vi "AluFlon Calibration.vi"() -> ()   [LabVIEW 2020]
uses:
  <vilib>/Instr/_visa.llb/VISA Find Search Mode.ctl
  <vilib>/Utility/miscctls.llb/LVRangeTypeDef.ctl
  de5aae1c-766f-4be6-99a3-fd4ec51816d1.vi
  444d9fc6-818c-47ea-bc58-0d0404dcb872.vi
  b5a75377-d0a3-43d6-8795-20c953c640ae.vi
  d5915287-11e6-429c-9896-de3842618b98.vi
  0cc29e98-fdb5-409f-a0e8-e594b8d976c3.vi
  0322f161-1cbb-43ba-a316-90f580a35a69.vi
  6005b055-fe01-43f0-bd4e-c0c49bb95745.vi
  ecbb4e81-cdd6-4c90-bb4c-f1c9c07fb26c.vi
  1a033c88-510c-45da-922e-66e902a61d4e.vi
  93b92521-9e16-4e93-a709-63335b20948f.vi
  31527b8b-dd2e-4aef-8780-3661b63cca63.vi
  b0d12dfb-2fe3-4095-91e7-f81a6dcb1a5e.vi
  c511048d-5316-4b7a-a317-28d3a9e40be0.vi
  e6c7d1cb-2e94-4559-8f57-83b39ddeefc4.vi
  0a39aaed-6fe6-4517-8bcb-3b5a94f10ea5.vi
  26b90bb2-1f84-4233-ae15-16fa66b975c9.vi
  89507e17-66a2-42ab-9a6b-fa3baa268747.vi
  6f735820-b968-40fe-8dcc-9caa75eabf9b.vi
  379c9800-c512-4a9e-8fef-dcae08926fd9.vi
  6bee6147-41c9-44c0-82a1-e9b70bc37061.vi
  dbb8d4b4-432b-4aa2-b5ee-fb03dd486db5.vi
  9e6f70b0-763e-423b-96ef-59fb8772dfa3.vi
  9a42ad8e-034c-4bb5-99e1-dddd59a1f9b6.vi
  3a4bb5ac-5c5c-4d63-87bf-9b8807b4be2b.vi
  a7842cd6-eb29-4009-89cc-97ffd3691122.vi
  a0a268c4-e710-4790-b893-111d5180be5d.vi
  66df6cea-0bd2-48ae-885a-3d43a00be0e6.vi
  87e030aa-6b8c-4722-a122-ccb5b3d7d58b.vi
  107db427-7959-46f3-9e7b-819df6104af8.vi
  de5aae1c-766f-4be6-99a3-fd4ec51816d1.vi/393b2312-c94a-42b8-a7f2-b1ce51657457.vi
  444d9fc6-818c-47ea-bc58-0d0404dcb872.vi/393b2312-c94a-42b8-a7f2-b1ce51657457.vi
  ecbb4e81-cdd6-4c90-bb4c-f1c9c07fb26c.vi/393b2312-c94a-42b8-a7f2-b1ce51657457.vi
  1a033c88-510c-45da-922e-66e902a61d4e.vi/393b2312-c94a-42b8-a7f2-b1ce51657457.vi
  93b92521-9e16-4e93-a709-63335b20948f.vi/393b2312-c94a-42b8-a7f2-b1ce51657457.vi
  31527b8b-dd2e-4aef-8780-3661b63cca63.vi/393b2312-c94a-42b8-a7f2-b1ce51657457.vi
  b0d12dfb-2fe3-4095-91e7-f81a6dcb1a5e.vi/393b2312-c94a-42b8-a7f2-b1ce51657457.vi
  c511048d-5316-4b7a-a317-28d3a9e40be0.vi/393b2312-c94a-42b8-a7f2-b1ce51657457.vi
  e6c7d1cb-2e94-4559-8f57-83b39ddeefc4.vi/393b2312-c94a-42b8-a7f2-b1ce51657457.vi
  0a39aaed-6fe6-4517-8bcb-3b5a94f10ea5.vi/393b2312-c94a-42b8-a7f2-b1ce51657457.vi
  26b90bb2-1f84-4233-ae15-16fa66b975c9.vi/393b2312-c94a-42b8-a7f2-b1ce51657457.vi
  89507e17-66a2-42ab-9a6b-fa3baa268747.vi/393b2312-c94a-42b8-a7f2-b1ce51657457.vi
  6f735820-b968-40fe-8dcc-9caa75eabf9b.vi/393b2312-c94a-42b8-a7f2-b1ce51657457.vi
  a0a268c4-e710-4790-b893-111d5180be5d.vi/393b2312-c94a-42b8-a7f2-b1ce51657457.vi
  <vilib>/NI Modbus.llb/MB Serial Master Query (poly).vi
  SubVI/MB Serial Master Query Write Single Register (poly).vi
  <vilib>/Utility/file.llb/Write Delimited Spreadsheet (string).vi
  <vilib>/Utility/miscctls.llb/LVStringsAndValuesArrayTypeDef_U16.ctl
panel:
  out "ConnectionFlag":bool=TRUE
  out "Blank Bottom":bool
  in  "visibleArray":bool[](array[boolean])
  in  "ClearTGraph 2":bool caption="Clear"
  in  "Dirt Calibr":bool caption="IRTimeSet"
  in  "ServiceWin":bool
  in  "file path (dialog if empty)":path
  out "Blank Top":bool
  out "FirmW":u16
  out "Serial":u16
  out "CC3":bool
  out "CC2":bool
  out "CC1":bool
  out "ConnectionStatus":bool=TRUE
  out "Critical Temp":bool
  out "Err Temp Ch":bool
  out "Err Press Ch":bool
  out "find list":string[](array[string])
  in  "Tab Control 2":enum32{"Page 1", "Page 2"}(tab)
  out "Cluster":T1
  in  "Config":bool
  out "error out":errorcluster={"status"=TRUE, "code"=0, "source"=""}
  out "VISA resource name":refnum<visa-resource-name>
  in  "Tab Control":T2(tab)
  in  "Частота опроса":i32=500 min=1 max=255 step=1
  in  "Update":bool
  in  "Порт":u16(ring)
  in  "BAUD":u16(ring)=9600 items=["1200"=1200, "2400"=2400, "4800"=4800, "9600"=9600, "19200"=19200, "38400"=38400]
  in  "Адрес датчика":u16=1 min=1 max=255 step=1
  in  "Connect":bool
  in  "DisconnectBtn":bool
  in  "CalibValue":sgl
  in  "SavePointCal 2":bool
  in  "CalPointN":u16(ring) items=["Температура", "Давление"]
  out "Temp/Press":cluster{"Pressure":sgl, "Reduced Pressure":sgl}(graph)
  in  "Momentary Autoscale":bool
  out "Temp meas":string
  out "Pressure meas 2":string
  out "Pressure meas":string
  in  "showReducedPressure":bool=TRUE
  in  "showTemp":bool=TRUE
  in  "showPressure":bool=TRUE
  out "Temperature":sgl caption="Температура" format="%.3g"
  out "Reduced pressure":sgl caption="Приведенное давление" format="%.3g"
  out "Destiny":sgl caption="Плотность" format="%.3g"
  out "Pressure":sgl caption="Давление" format="%.3g"
  out "Graph":T3(graph)
  in  "showDestiny":bool=TRUE
  in  "Load Backup":bool
  in  "Create Backup":bool
  in  "ChangeTempUnits":bool
  in  "Temp units new":dbl(ring)=1.0 caption="Температура в" items=["°С"=1.0, "F"=32.0, "K"=273.5]
  in  "Temp units":dbl(ring)=1.0 caption="Температура в" items=["°С"=1.0, "F"=32.0, "K"=273.5]
  in  "ChangePressureUnits":bool
  in  "Pressure units new":T4(ring) caption="Давление в"
  in  "Pressure units":T4(ring) caption="Давление в"
  out "File Path":path caption="Файл журнала"
  in  "SaveTLog?":bool caption="Лог?"
  in  "NewDestiny":sgl=1.0 min=1 max=255 step=1
  in  "Change Destiny":bool
  out "Плотность":sgl=1.0 min=1 max=255 step=1
  in  "modeChange":bool
  in  "Mode":u16(ring)=1 items=["Пользователь"=1, "Инженер"=2]
  out "Режим работы":u16(ring)=1 items=["Пользователь"=1, "Инженер"=2, ""=0]
  out "Адрес":u16=1 min=1 max=255 step=1
  in  "NewSlave":u16=1 min=1 max=255 step=1
  in  "ChangeSlaveAdress":bool
  in  "Tab Service":T5(tab)
  in  "Visible5":bool caption="Лог?"
  in  "Visible4":bool caption="Лог?"
  in  "Visible3":bool caption="Лог?"
  in  "Visible2":bool caption="Лог?"
  in  "FitRawGraph":bool caption="Clear"
  in  "ClearRAWGraph":bool caption="Clear"
  in  "ClearTGraph":bool caption="Clear"
  out "Sensor":T6(graph)
  out "Temp/Press":cluster{"Pressure":sgl, "Reduced Pressure":sgl}(graph)
  out "Gas Detected":u32(colorbox)
  out "ThermalDrift":u32(colorbox) caption="Thermal drift"
  out "Impact":u32(colorbox) caption="Mechanical"
  out "Starting":u32(colorbox)
  in  "DataType":u16(ring) items=["PID filter"=3, "Normalized"=2, "Averaged"=1, "RAW"=0]
  in  "Visible1":bool caption="Лог?"
  in  "Firmware":i32=1930 min=1 max=12 step=1
  in  "Setfirm":bool
  in  "SetSerialN":bool
  in  "SerialNumber":i32=1930 min=1 max=12 step=1
  out "heatLowLimRd_":i32=110 min=1 max=12 step=1
  in  "heatLowLimW":bool caption="SET"
  in  "heatLowLimSP":i32=1930 min=1 max=12 step=1
  out "heatUpLimRd_":i32=110 min=1 max=12 step=1
  in  "heatUpLimW":bool caption="SET"
  in  "heatUpLimSP":u16=1990 min=1 max=12 step=1
  out "TaskTimeRead":i32 min=1 max=12 step=1
  in  "TaskSet":bool caption="TaskTime"
  in  "TaskTime":i32=900 min=1 max=12 step=1
  out "IR Time R":i32=110 min=1 max=12 step=1
  in  "IRSetBtn":bool caption="SET"
  in  "IR Time":i32=110 min=1 max=12 step=1
  in  "WirenSet":bool
  in  "WirenSetMode":bool caption="Коэф. загрязнения\nx100"
  out "WirenMode_":bool
  in  "DirtKoefRSet":i32=100 min=1 max=12 step=1
  in  "DirtKoefBtnW":bool caption="Коэф Загряз"
  out "DirtKoefR":i32=220 min=1 max=12 step=1
  in  "DirtKoefRSet 2":u16=500 min=1 max=12 step=1
  in  "LowSignalBtnSet":bool caption="Коэф Загряз"
  out "LowLevelRead":u16=220 min=1 max=12 step=1
  in  "Выкл":bool
  in  "HeaterBreakerSet":bool=TRUE
  out "HeatRead":bool
  out "ZeroShifr":u8 min=1 max=12 step=1
  in  "ZeroShiftSet":u16=5 min=1 max=12 step=1
  in  "ZeroShiftSetBtn":bool caption="Смещение \nнуля"
  in  "ContaminSet":bool caption="Коэф. загрязнения\nx100"
  in  "ContaminantSetPoint":i16=225 min=1 max=12 step=1
  out "DirtChRead":i16 min=1 max=12 step=1
  out "Месяц":i8=5
  out "Год":i8=2
  in  "Month":u8=3 min=1 max=12 step=1
  in  "Year":u8=17 max=99 step=1
  in  "VerificationBtnSet":bool caption="Год"
  in  "Err 6":bool=TRUE
  in  "Err 5":bool=TRUE
  in  "Err 7":bool=TRUE
  in  "Err 4":bool=TRUE
  in  "Err 3":bool=TRUE
  in  "Err 2":bool=TRUE
  in  "Err 1":bool=TRUE
  in  "Err 0":bool=TRUE
  in  "BlockErrorSet":bool caption="W"
  in  "SetGain":bool caption="TaskTime"
  in  "OK Button":bool
  out "gainLED":bool
  out "MagnetRead":bool
  in  "MagnetSP":bool=TRUE
  in  "MagnetWrite":bool
  in  "thermoGradientSP_Set":bool caption="Коэф. загрязнения\nx100"
  in  "thermoGradientSP":i16=225 min=1 max=12 step=1
  out "thermoGradientS_R":i16 min=1 max=12 step=1
  in  "getCorner":bool caption="Год"
  out "spanZ":i16=2
  out "cornerGas":i16=2
  out "cornerRef":i16=2
  in  "gasNoise_set":bool caption="Коэф. загрязнения\nx100"
  in  "gasNoiseSP":i16=225 min=1 max=12 step=1
  out "gasNoiseSP_R":i16 min=1 max=12 step=1
  in  "refNoiseSP_set":bool caption="Коэф. загрязнения\nx100"
  in  "refNoiseSP":i16=225 min=1 max=12 step=1
  out "refNoiseSP_R":i16 min=1 max=12 step=1
  in  "stablePirSP_Set":bool caption="Коэф. загрязнения\nx100"
  in  "stablePirSP":i16=225 min=1 max=12 step=1
  out "stablePirSP_R":i16 min=1 max=12 step=1
  out "XY graph 4":cluster{i32[], i32[]}(graph)
  in  "ThermoTableBtnW":bool caption="IRTimeSet"
  in  "SaveTermo":bool caption="IRTimeSet"
  out "Array INT Temp":i32[][](array[numeric])
  in  "ReadTermoData":bool caption="IRTimeSet"
  out "XY graph 3":cluster{i32[], i32[]}(graph)
  in  "WriteCalibrData":bool caption="IRTimeSet"
  in  "SaveGasCalibr":bool caption="IRTimeSet"
  in  "ReadCalData":bool caption="IRTimeSet"
  out "Array INT":i32[][](array[numeric])
  out "XY graph 2":T7(graph)
  out "ResetTi":dbl(slide) scale=0.0..11.0
  in  "Перезагрузка":bool caption="IRTimeSet"
  in  "Заводские\nнастройки":bool caption="IRTimeSet"
  in  "DispB":bool
  in  "CalibrB":bool
  in  "Setngs485":bool=TRUE
  in  "Mode":enum16{"RTU", "ASCII"}(ring)
  out "Lost":i16
  # "Подключение"
  # "ИГАС DM-910"
  # "Серийный №"
  # "Прошивка"
  # "Калибровка нуля"
  # "Шаг 1. \nВыберите калибруемый параметр"
  # "Шаг 2.\nВведите нужное значение"
  # "Шаг 3.\nСохраните результаты процедуры"
  # "Применить ?"
  # "г/л"
  # "Новые настройки"
  # "Текущие настройки"
  # "Журнал показаний:"
  # "Оптика"
  # "Дельта"
  # "Выход газ"
  # "Выход реф"
  # "Сигнал газ"
  # "Сигнал реф"
  # "Текущее\nзначение"
  # "Текущее\nзначение"
  # "Запись"
  # "Запись"
  # "Параметр"
  # "Параметр"
  # "Внешнее реле"
  # "ИК Импульс"
  # "Уровень\nзагрязнений"
  # "Время цикла"
  # "Предел нагрева\nВерх"
  # "Предел нагрева\nниз"
  # "Нагреватель"
  # "Уровень\nаварийного\nсигнала"
  # "Серийный\nномер"
  # "Поправка \nзагрязнений"
  # "Прошивка"
  # "Усиление"
  # "Магнитная\nкалибровка"
  # "Блокировка ошибок"
  # "Текущее\nзначение"
  # "Запись"
  # "Параметр"
  # "Стартовый шум"
  # "Градиент\nопорного канала"
  # "Градиент \nгазового канала"
  # "Градиент \nтемпературы"
  # "Термостабилизация"
  # "Сохранить"
  # "Записать"
  # "Прочитать"
  # "Калибровка по газу"
  # "Прочитать"
  # "Записать"
  # "Сохранить"
  # "0"
  # "min"
  # "1"
  # "max"
  # "2"
  # "mode"
  # "3"
  # "peakAddr"
  # "4"
  # "max-min"
  # "5"
  # "peaks"
  # "6"
  # "run1"
  # "7"
  # "run2"
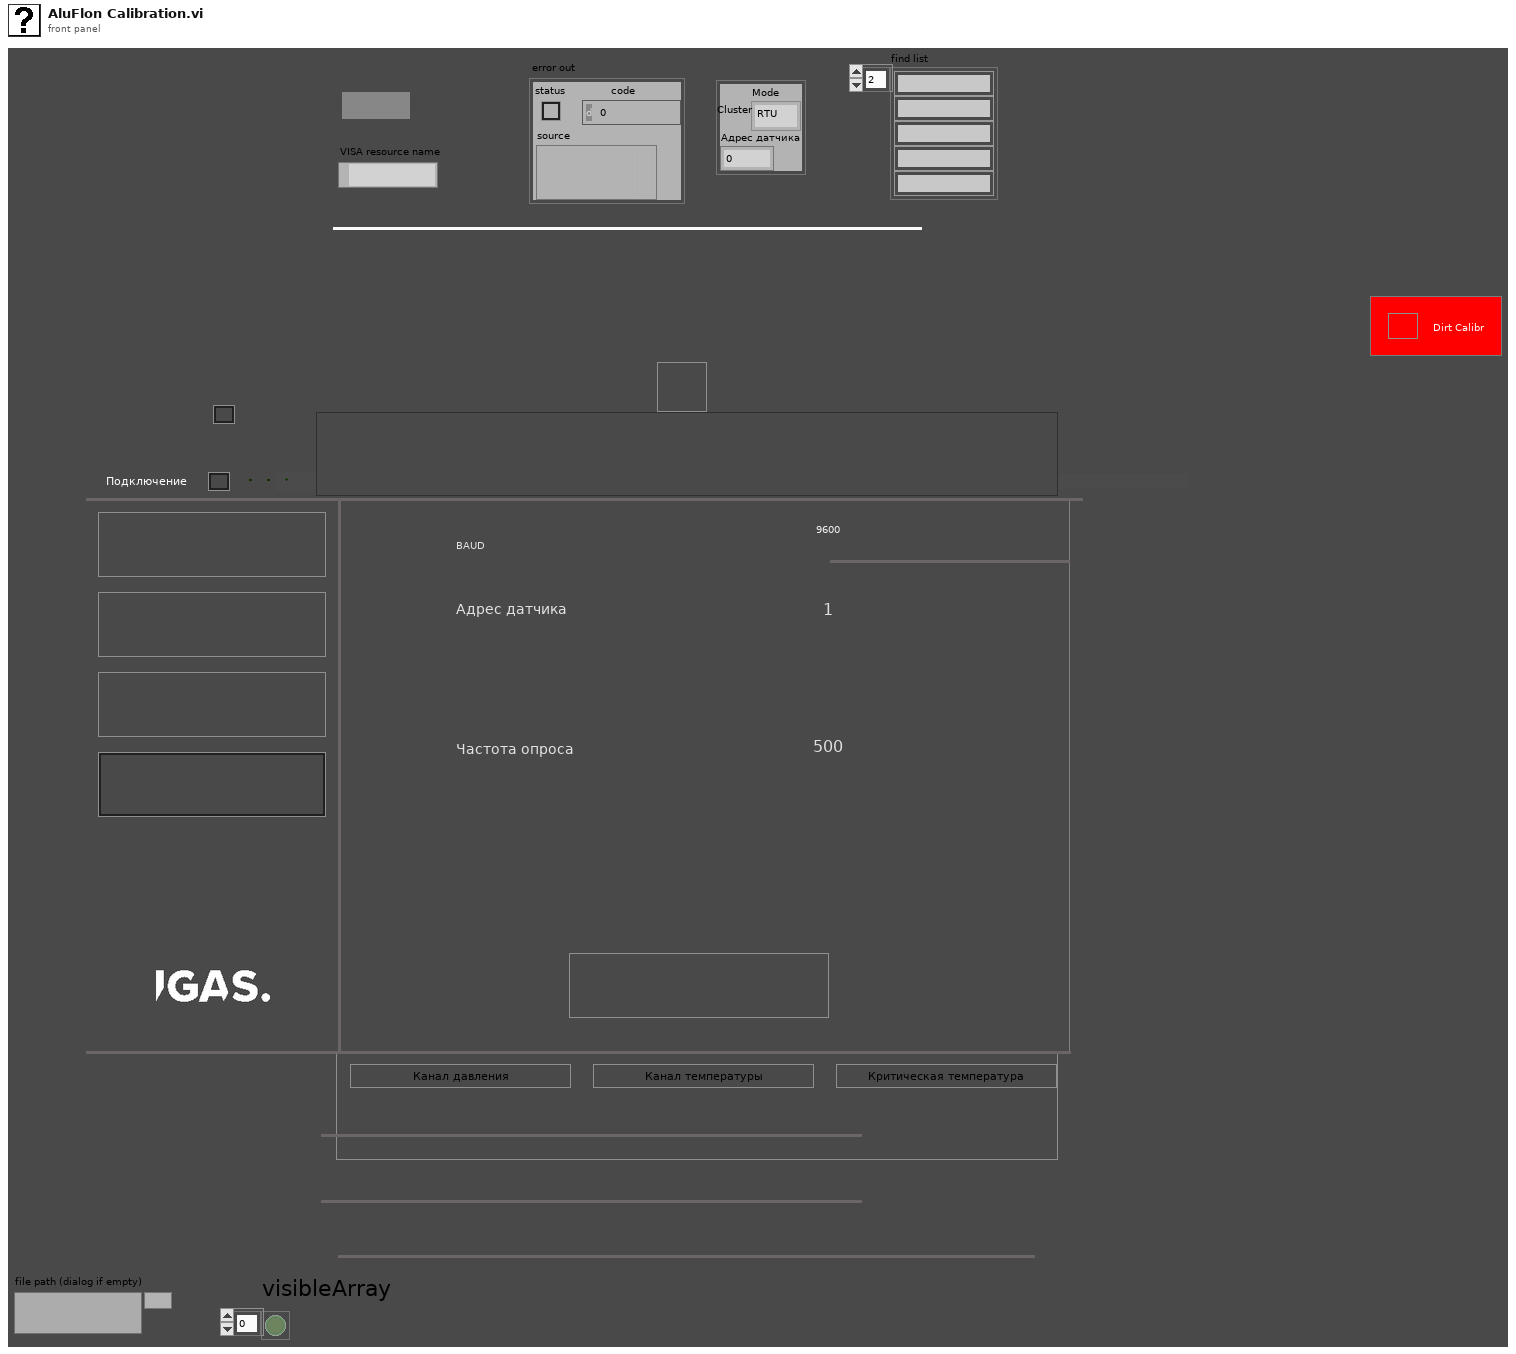
[diagram p1: front panel]
types:
  T1 = cluster{"Mode":enum16{"RTU", "ASCII"}, "Адрес датчика":u16}
  T2 = enum32{"Settings", "Calibration", "Display", "Config", "Service"}
  T3 = cluster{"Reduced Pressure":sgl, "Pressure":sgl, dbl, "Destiny":sgl}
  T4 = enum16{"кг/см2", "мм рт. ст.", "гПа", "кПа", "МПа", "мм вод. ст.", "psi"}
  T5 = enum32{"Графики", "Сервисные настройки", "Фильтр", "Термо компенсация", "Газовая калибровка", "Команды", "Debug"}
  T6 = cluster{"Numeric":dbl, "Numeric":dbl, "Numeric":dbl, "Numeric":dbl, "Numeric":dbl}
  T7 = cluster{"Holding Registers":u16[], "Holding Registers":u16[]}[]
  T8 = cluster{"Reduced Pressure":sgl, "Pressure":sgl, "Temperature":sgl, "Destiny":sgl}[]
  T9 = enum32{"Settings", "Calibration", "Display", "Config"}
  T10 = enum8{"Enabled", "Disabled", "Disabled and Grayed Out"}
  T11 = enum32{"Settings", "Calibration", "Display", "Config", "Temperature Tuning"}
  T12 = typedef "LVStringsAndValuesArrayTypeDef_U16.ctl" = cluster{"String":string, "Value":u16}[]
  T13 = typedef "LVRangeTypeDef.ctl" = cluster{"Minimum":dbl, "Maximum":dbl, "Increment":dbl, "Minor Increment":dbl, "Start":dbl}
  T14 = typedef "VISA Find Search Mode.ctl" = u32
  T15 = cluster{"Pressure":sgl, "Reduced Pressure":sgl}[]
  T16 = cluster{"Numeric":dbl, "Numeric":dbl, "Numeric":dbl, "Numeric":dbl, "Numeric":dbl}[]
  T17 = cluster{"Pressure":sgl, "Temperature":sgl, "Reduced Pressure":sgl, "Destiny":sgl, "Error Pressure Ch":bool, "Error Temp Ch":bool, "Critical Temp":bool}
  T18 = cluster{"Mode":enum16{"RTU", "ASCII"}, "Новый адрес датчика":u16}
  T19 = cluster{"Mode":enum16{"RTU", "ASCII"}, "Numeric":u16}
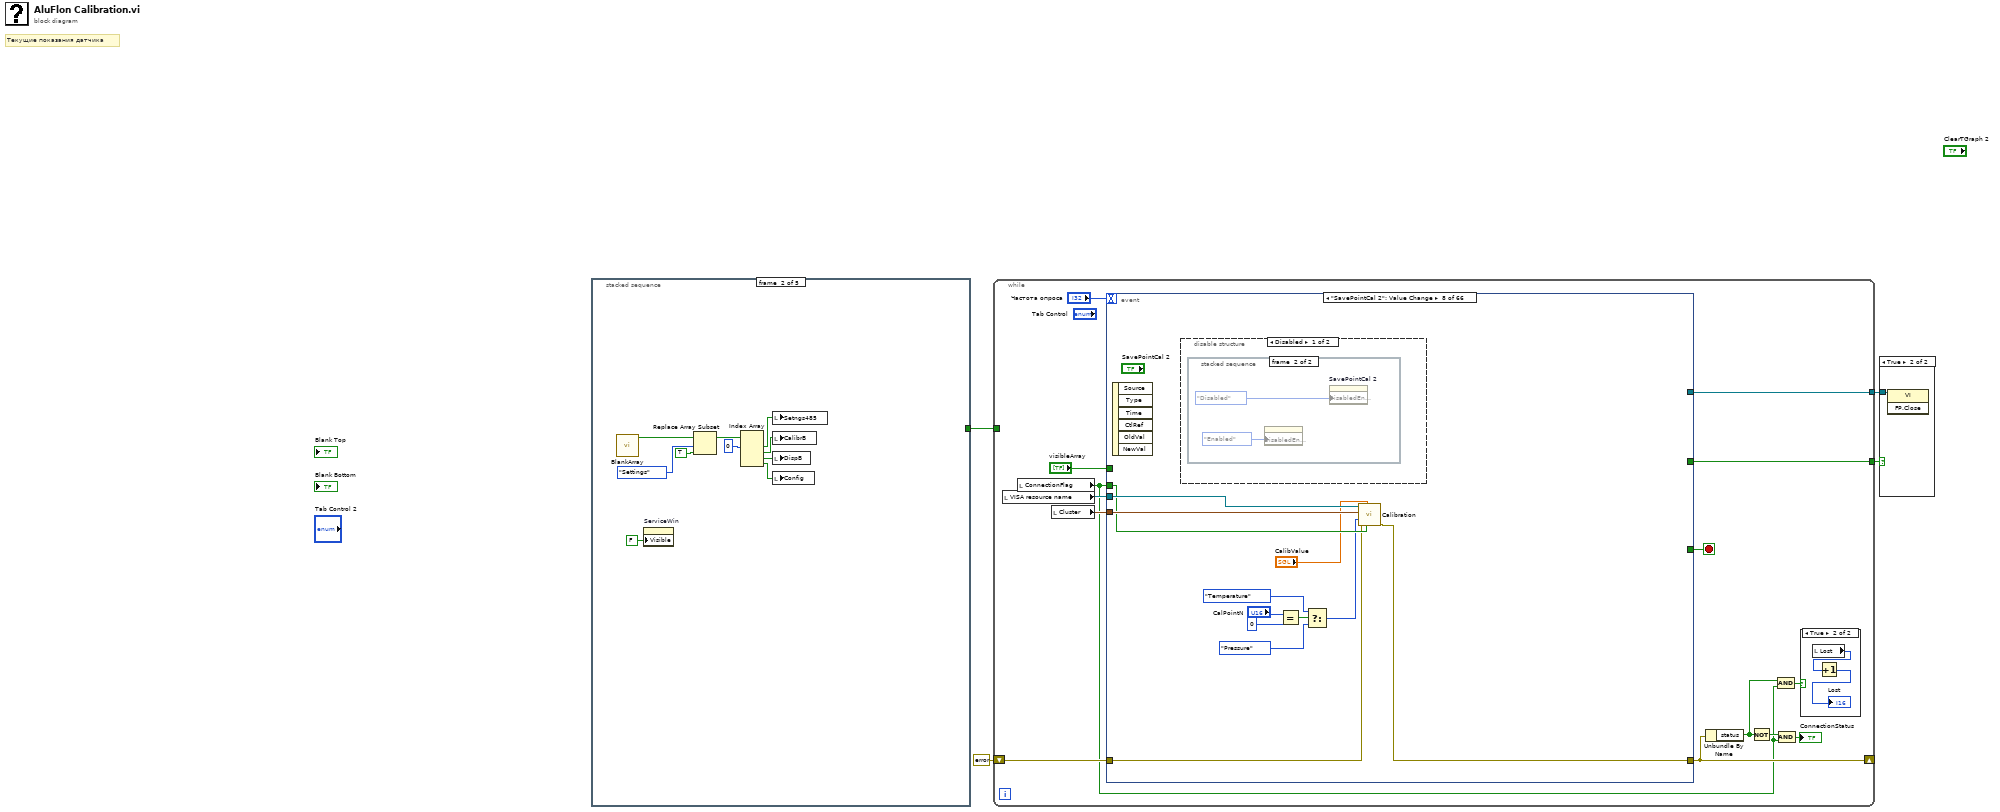
[diagram p0: block diagram]
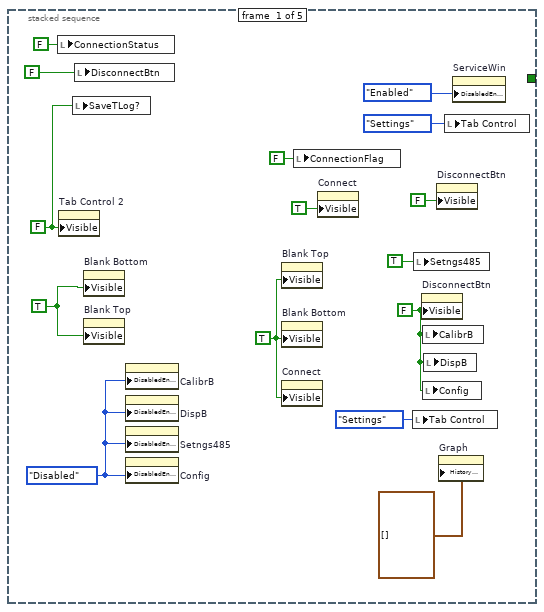
[diagram p3: hidden frame]
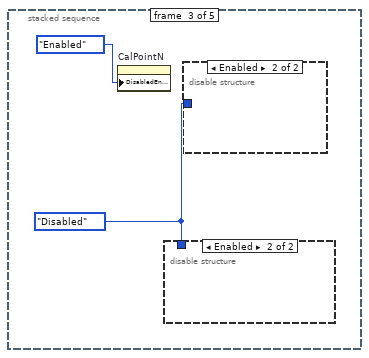
[diagram p4: hidden frame]
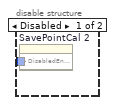
[diagram p5: hidden frame]
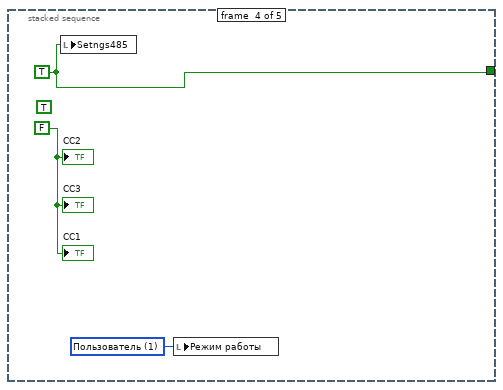
[diagram p7: hidden frame]
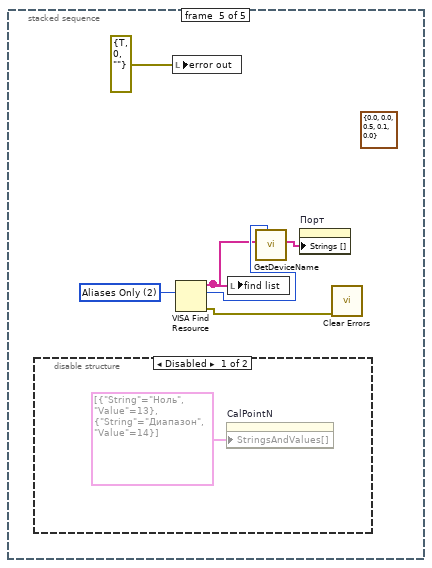
[diagram p8: hidden frame]
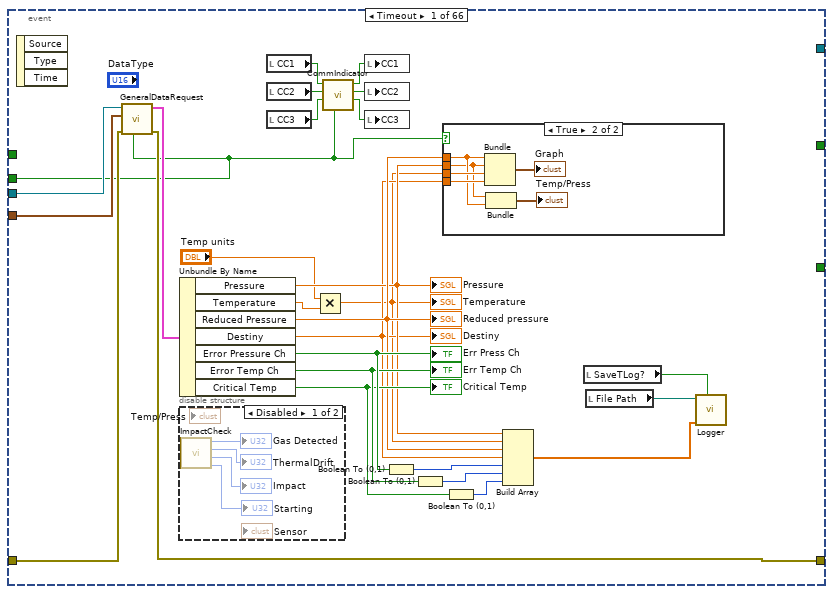
[diagram p11: hidden frame]
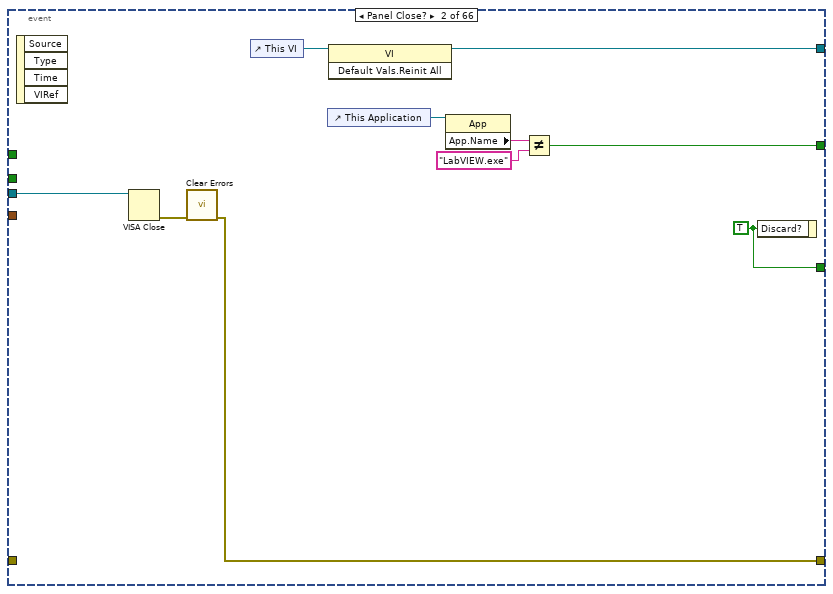
[diagram p14: hidden frame]
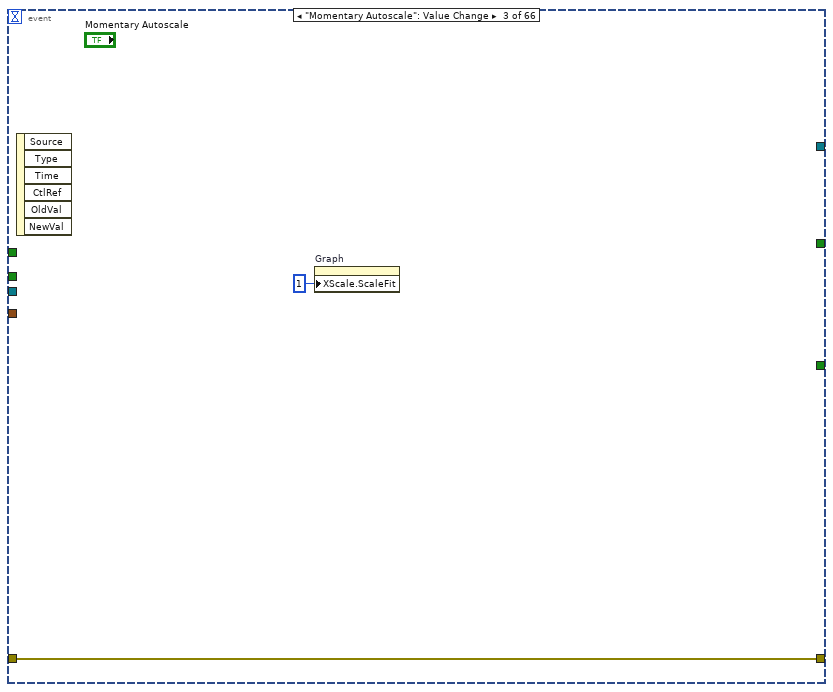
[diagram p15: hidden frame]
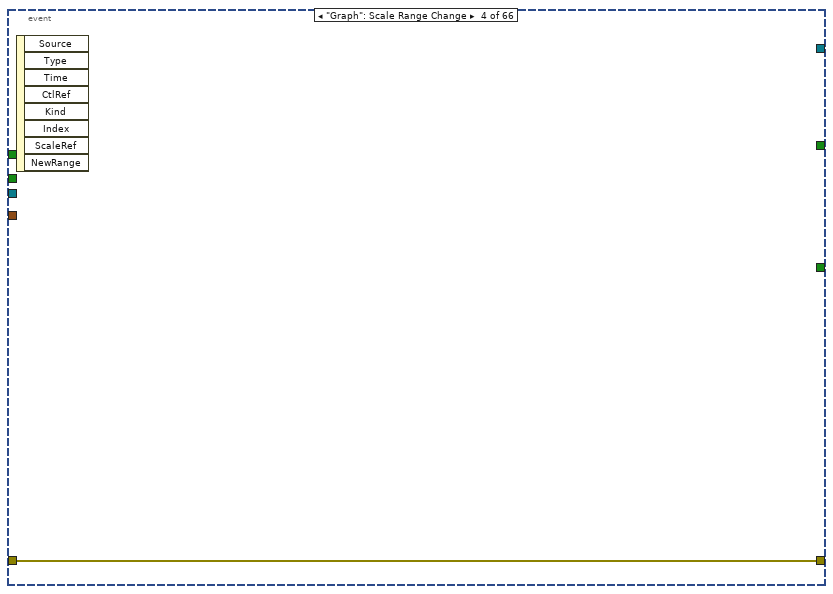
[diagram p16: hidden frame]
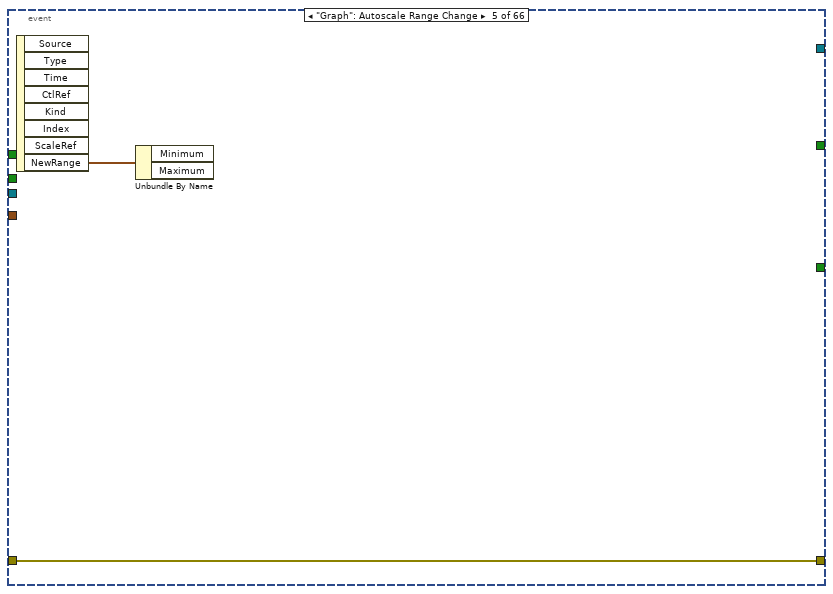
[diagram p17: hidden frame]
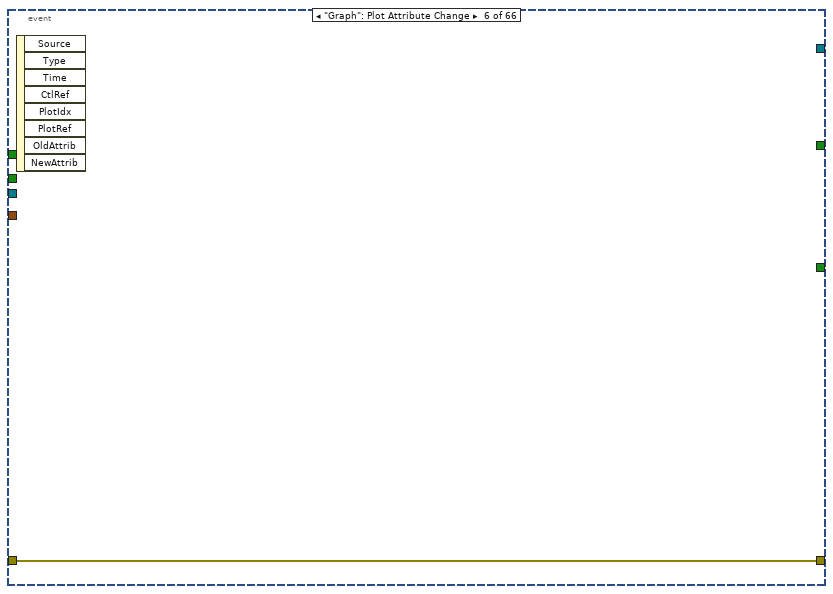
[diagram p18: hidden frame]
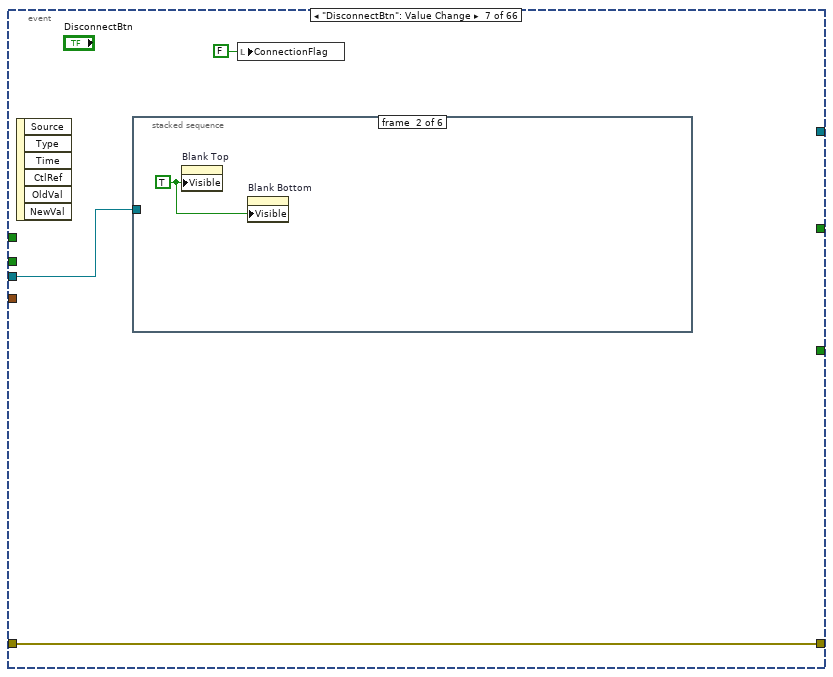
[diagram p19: hidden frame]
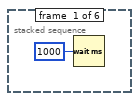
[diagram p20: hidden frame]
diagram:
  # "Текущие показания датчика"
  n1 = stacked-sequence {
    tunnel: [_ _ _ w35 _] -> w4
    frame #0 {
      w9 = FALSE
      w10 = TRUE
      w7 = T10."Disabled" ("Disabled")
      w16 = TRUE ("Visible")
      w18 = FALSE ("Visible")
      n2 = local write "ConnectionStatus"(FALSE ("ConnectionStatus")) -> ()
      n3 = property on="Tab Control 2" class="TabCtl (strict)"("Visible"=w18) -> ()  [unwired: 2 in, 2 out]
      n4 = local write "SaveTLog?"(w18) -> ()
      n5 = local write "DisconnectBtn"(FALSE ("DisconnectBtn")) -> ()
      n6 = property on="Blank Bottom" class="Bool (strict)"("Visible"=w16) -> ()  [unwired: 2 in, 2 out]
      n7 = property on="Blank Top" class="Bool (strict)"("Visible"=w16) -> ()  [unwired: 2 in, 2 out]
      n8 = property on="CalibrB" class="Bool (strict)"("DisabledEnum"=w7) -> ()  [unwired: 2 in, 2 out]
      n9 = property on="DispB" class="Bool (strict)"("DisabledEnum"=w7) -> ()  [unwired: 2 in, 2 out]
      n10 = property on="Setngs485" class="Bool (strict)"("DisabledEnum"=w7) -> ()  [unwired: 2 in, 2 out]
      n11 = property on="Config" class="Bool (strict)"("DisabledEnum"=w7) -> ()  [unwired: 2 in, 2 out]
      n12 = property on="Blank Top" class="Bool (strict)"("Visible"=w10) -> ()  [unwired: 2 in, 2 out]
      n13 = property on="Blank Bottom" class="Bool (strict)"("Visible"=w10) -> ()  [unwired: 2 in, 2 out]
      n14 = property on="Connect" class="Bool (strict)"("Visible"=w10) -> ()  [unwired: 2 in, 2 out]
      n15 = local write "ConnectionFlag"(FALSE ("ConnectionFlag")) -> ()
      n16 = property on="Connect" class="Bool (strict)"("Visible"=TRUE) -> ()  [unwired: 2 in, 2 out]
      n17 = local write "Tab Control"(T2."Settings" ("Tab Control")) -> ()
      n18 = local write "Setngs485"(TRUE ("CalibrB")) -> ()
      n19 = property on="DisconnectBtn" class="Bool (strict)"("Visible"=w9) -> ()  [unwired: 2 in, 2 out]
      n20 = local write "CalibrB"(w9) -> ()
      n21 = local write "Config"(w9) -> ()
      n22 = local write "DispB"(w9) -> ()
      n23 = property on="DisconnectBtn" class="Bool (strict)"("Visible"=FALSE) -> ()  [unwired: 2 in, 2 out]
      n24 = property on="Graph" class="WFChart (strict)"("History Data"=T8 []) -> ()  [unwired: 2 in, 2 out]
      n25 = local write "Tab Control"(T9."Settings" ("Tab Control")) -> ()
      n26 = property on="ServiceWin" class="Bool (strict)"("DisabledEnum"=T10."Enabled" ("Disabled")) -> ()  [unwired: 2 in, 2 out]
    }
    frame #1 {
      n27 = call "BlankArray.vi"() -> ("Array"=w23:bool[])  [unwired: 11 in]
      n28 = property on="ServiceWin" class="Bool (strict)"("Visible"=FALSE) -> ()  [unwired: 2 in, 2 out]
      n29 = Replace Array Subset(array=w23, new element=TRUE ("SettingsB"), index=T11."Settings" ("Tab Control")) -> (w24:bool[])
      n30 = Index Array(array=w24, index #1=0 ("index")) -> (element #1=w27:bool, element #2=w26:bool, element #3=w21:bool, element #4=w22:bool)  [unwired: 3 in]
      n31 = local write "Setngs485"(w27) -> ()
      n32 = local write "CalibrB"(w26) -> ()
      n33 = local write "DispB"(w21) -> ()
      n34 = local write "Config"(w22) -> ()
    }
    frame #2 {
      w30 = T10."Disabled" ("Disabled")
      n35 = property on="CalPointN" class="Ring (strict)"("DisabledEnum"=T10."Enabled" ("Disabled")) -> ()  [unwired: 2 in, 2 out]
      n36 = disable-structure shown="Enabled" {
        disable-tunnel: w30 -> [w33 _]
        frame Disabled {
        }
        frame Enabled {
        }
      }
      n37 = disable-structure shown="Enabled" {
        disable-tunnel: w30 -> [w32 _]
        frame Disabled {
          n38 = property on="SavePointCal 2" class="Bool"("DisabledEnum"=w32) -> ()  [unwired: 2 in, 2 out]
        }
        frame Enabled {
        }
      }
    }
    frame #3 {
      (unwired) TRUE ("ConnectionStatus")
      w34 = u16 1 items=["Пользователь"=1, "Инженер"=2, ""=0] ("Режим работы")
      w35 = TRUE ("ConnectionStatus")
      w36 = FALSE ("ConcentrationBTn")
      n39 = local write "Setngs485"(w35) -> ()
      n40 = local write "Режим работы"(w34) -> ()
      "CC1" <- w36
      "CC2" <- w36
      "CC3" <- w36
    }
    frame #4 {
      (unwired) T13 {"Minimum"=0.0, "Maximum"=0.0, "Increment"=0.5, "Minor Increment"=0.1, "Start"=0.0} ("Y Scale.Range")
      w42 = T14 2 items=["Canonical Names Only"=0, "Aliases Only"=2, "Include Matching Aliases"=3, "Include All Aliases"=4] ("Search Mode")
      n41 = disable-structure shown="Disabled" {
        frame Disabled {
          n42 = property on="CalPointN" class="Ring (strict)"("StringsAndValues[]"=T12 [{"String"="Ноль", "Value"=13}, {"String"="Диапазон", "Value"=14}] ("Strings And Values []")) -> ()  [unwired: 2 in, 2 out]
        }
        frame Enabled {
        }
      }
      n43 = local write "error out"(errorcluster {"status"=TRUE, "code"=0, "source"=""} ("error out")) -> ()
      n44 = VISA Find Resource(10:w42) -> (0:w37:errorcluster, 2:w39:u32, 3:w38:string[])  [unwired: 2 in]
      n45 = local write "find list"(w38) -> ()
      n46 = call "GetDeviceName.vi"("PortQuantity"=w39, "Input"=w38) -> ("Output"=w40:string[])  [unwired: 9 in]
      n47 = property on="Порт" class="Ring (strict)"("Strings []"=w40) -> ()  [unwired: 2 in, 2 out]
      n48 = call <vilib>:"Clear Errors.vi"("error in (no error)"=w37) -> ()  [unwired: 5 in, 2 out]
    }
  }
  n49 = while {
    tunnel: w4 -> [_]
    shift-right: [w53] -> _
    shift-left: errorcluster {"status"=FALSE, "code"=0, "source"=""} ("error out") -> [w51]
    tunnel: [w48] -> w2
    tunnel: [w47] -> w1
    stop <- w49 stop-if-true
    n50 = local read "VISA resource name"() -> (w56:refnum<visa-resource-name>)
    n51 = local read "ConnectionFlag"() -> (w45:bool)
    n52 = local read "Cluster"() -> (w57:T1)
    n53 = event shown="[7] \"SavePointCal 2\": Value Change" {
      selector: _ -> [_ _ _ _ _ _ _ _ _ _ _ _ _ _ _ _ _ _ _ _ _ _ _ _ _ _ _ _ _ _ _ _ _ _ _ _ _ _ _ _ _ _ _ _ _ _ _ _ _ _ _ _ _ _ _ _ _ _ _ _ _ _ _ _ _ _]
      dyn-events: _ -> [_ _ _ _ _ _ _ _ _ _ _ _ _ _ _ _ _ _ _ _ _ _ _ _ _ _ _ _ _ _ _ _ _ _ _ _ _ _ _ _ _ _ _ _ _ _ _ _ _ _ _ _ _ _ _ _ _ _ _ _ _ _ _ _ _ _]
      timeout: "Частота опроса" -> [_ _ _ _ _ _ _ _ _ _ _ _ _ _ _ _ _ _ _ _ _ _ _ _ _ _ _ _ _ _ _ _ _ _ _ _ _ _ _ _ _ _ _ _ _ _ _ _ _ _ _ _ _ _ _ _ _ _ _ _ _ _ _ _ _ _]
      tunnel: w56 -> [w78 w106 _ _ _ _ w114 w142 _ _ _ _ _ w173 _ _ _ _ _ w236 w244 w251 w265 w272 w295 _ w307 _ _ _ _ _ _ _ _ w369 w377 w384 w392 w400 w407 w415 w430 w439 w455 w462 w469 w476 w483 _ _ w537 w544 w550 w569 w590 _ w603 w614 w619 w633 _ _ w649 w661 w674]
      tunnel: w57 -> [w77 _ _ _ _ _ _ w141 _ _ _ _ _ w171 _ _ _ _ _ w234 w242 w250 w262 w271 w294 _ w306 _ _ _ _ _ _ _ _ w368 w376 w383 w391 w399 w406 w414 w431 w440 w456 w463 w470 w477 w484 _ _ w538 w543 w551 w568 w589 _ w602 w613 w620 w632 _ _ w647 w660 w675]
      tunnel: "visibleArray" -> [_ _ _ _ _ _ _ _ _ _ _ _ _ _ _ _ _ _ _ _ _ _ _ _ _ _ _ _ _ w335 w342 w348 w354 w360 _ _ _ _ _ _ _ _ _ _ _ _ _ _ _ _ _ _ _ _ _ _ _ _ _ _ _ _ _ _ _ _]
      tunnel: w45 -> [w60 _ _ _ _ _ _ w140 _ _ _ _ _ w168 _ _ _ _ _ w231 w239 w247 w261 w268 w291 _ w304 _ _ _ _ _ _ _ _ w367 w374 w381 w388 w396 w403 w410 w418 w434 w452 w459 w466 w473 w480 _ _ w540 w545 w547 w556 w574 _ w601 w611 w616 _ _ _ _ w651 w672]
      tunnel: [w62 w97 w107 w109 w110 w112 w113 w139 w145 w154 w157 w160 w163 w167 w174 w185 w196 w207 w218 w230 w238 w246 w260 w267 w290 w296 w303 w310 w311 w333 w339 w345 w351 w357 w364 w366 w373 w380 w387 w395 w402 w409 w417 w433 w451 w458 w465 w472 w479 w485 w492 w539 w542 w546 w552 w573 w591 w599 w610 w615 w621 w637 w643 w645 w653 w671] -> w53
      tunnel: w51 -> [w61 _ w107 w109 w110 w112 w113 w137 w145 w154 w157 w160 w163 w166 w174 w185 w196 w207 w218 w229 w237 w245 w259 w266 w289 w296 w302 w310 w311 w333 w339 w345 w351 w357 w364 w365 w372 w379 w386 w394 w401 w408 w416 w432 w450 w457 w464 w471 w478 w485 w491 w536 w541 _ _ _ w591 _ _ _ _ w637 w643 _ _ w670]
      tunnel: [_ w104 _ _ _ _ _ _ _ _ _ _ _ _ _ _ _ _ _ _ _ _ _ _ _ _ _ _ _ _ _ _ _ _ _ _ _ _ _ _ _ _ _ _ _ _ _ _ _ _ _ _ _ _ _ _ _ _ _ _ _ _ _ _ _ _] -> w49
      tunnel: [_ w99 _ _ _ _ _ _ _ _ _ _ _ _ _ _ _ _ _ _ _ _ _ _ _ _ _ _ _ _ _ _ _ _ _ _ _ _ _ _ _ _ _ _ _ _ _ _ _ _ _ _ _ _ _ _ _ _ _ _ _ _ _ _ _ _] -> w48
      tunnel: [_ w98 _ _ _ _ _ _ _ _ _ _ _ _ _ _ _ _ _ _ _ _ _ _ _ _ _ _ _ _ _ _ _ _ _ _ _ _ _ _ _ _ _ _ _ _ _ _ _ _ _ _ _ _ _ _ _ _ _ _ _ _ _ _ _ _] -> w47
      event Timeout {
        n54 = event-data() -> ()  [unwired: 1 in, 3 out]
        n55 = call "GeneralDataRequest.vi"("Enable"=w60, "error in (no error)"=w61, "Cluster"=w77, "VISA Refnum in"=w78) -> ("error out"=w62:errorcluster, "Sensor data"=w76:T17)  [unwired: 6 in]
        n56 = Unbundle By Name(w76) -> ("Pressure"=w67:sgl, "Temperature"=w64:sgl, "Reduced Pressure"=w68:sgl, "Destiny"=w66:sgl, "Error Pressure Ch"=w75:bool, "Error Temp Ch"=w74:bool, "Critical Temp"=w73:bool)
        "Err Press Ch" <- w75
        "Err Temp Ch" <- w74
        "Critical Temp" <- w73
        "Pressure" <- w67
        "Destiny" <- w66
        "Reduced pressure" <- w68
        n57 = disable-structure shown="Disabled" {
          frame Disabled {
            n58 = call "ImpactCheck.vi"() -> ("Start"=→"Starting":u32, "Impact"=→"Impact":u32, "Thermal"=→"ThermalDrift":u32, "Gas Detected"=→"Gas Detected":u32)  [unwired: 8 in]
          }
          frame Enabled {
          }
        }
        n59 = local read "CC1"() -> (w86:bool)
        n60 = local read "CC2"() -> (w85:bool)
        n61 = local read "CC3"() -> (w84:bool)
        n62 = Multiply(x="Temp units", y=w64) -> (x*y=w65:dbl)
        "Temperature" <- w65
        n63 = call "CommIndicator.vi"("Allow"=w60, "In3"=w84, "In2"=w85, "In1"=w86) -> ("Out3"=w82:bool, "Out2"=w81:bool, "Out1"=w83:bool)  [unwired: 5 in]
        n64 = local write "CC1"(w83) -> ()
        n65 = local write "CC2"(w81) -> ()
        n66 = local write "CC3"(w82) -> ()
        n67 = Boolean To (0,1)(Boolean=w75) -> (0, 1=w70:i16)
        n68 = Boolean To (0,1)(Boolean=w74) -> (0, 1=w71:i16)
        n69 = case shown="True" w60 {
          tunnel: w68 -> [_ w89]
          tunnel: w67 -> [_ w88]
          tunnel: w65 -> [_ w92]
          tunnel: w66 -> [_ w91]
          frame False {
          }
          frame True {
            n70 = Bundle("Reduced Pressure"=w89, "Pressure"=w88, w92, "Destiny"=w91) -> (→"Graph":T3)  [unwired: 1 in]
            n71 = Bundle("Pressure"=w88, "Reduced Pressure"=w89) -> (→"Temp/Press":cluster{"Pressure":sgl, "Reduced Pressure":sgl})  [unwired: 1 in]
          }
        }
        n72 = Boolean To (0,1)(Boolean=w73) -> (0, 1=w72:i16)
        n73 = Build Array(w67, w65, w68, w66, w70, w71, w72) -> (w69:dbl[])
        n74 = local read "SaveTLog?"() -> (w80:bool)
        n75 = local read "File Path"() -> (w79:path)
        n76 = call "Logger.vi"("SaveLog?"=w80, "Input"=w69, "selected path in"=w79) -> ()  [unwired: 9 in]
      }
      event Panel Close? {
        w104 = TRUE ("Discard?")
        n77 = event-data() -> ()  [unwired: 1 in, 4 out]
        n78 = VISA Close(VISA resource name=w106) -> (error out=w105:errorcluster)  [unwired: 1 in]
        n79 = call <vilib>:"Clear Errors.vi"("error in (no error)"=w105) -> ("error out"=w97:errorcluster)  [unwired: 5 in, 1 out]
        n80 = control-ref of="This VI"() -> (w100:refnum<vi>)
        n81 = control-ref of="This Application"() -> (w102:refnum<vi>)
        n82 = invoke class="VI" method="Default Vals.Reinit All"(reference=w100) -> (reference out=w98:refnum<vi>)  [unwired: 2 in, 2 out]
        n83 = property class="App"(reference=w102) -> ("App.Name"=w103:string)  [unwired: 1 in, 2 out]
        n84 = Not Equal?(x=w103, y="LabVIEW.exe") -> (x != y?=w99:bool)
        n85 = event-data("Discard?"=w104) -> ()  [unwired: 1 in, 1 out]
      }
      event "Momentary Autoscale": Value Change {
        n86 = event-data() -> ()  [unwired: 1 in, 6 out]
        n87 = property on="Graph" class="WFChart (strict)"("XScale.ScaleFit"=u8 1 ("Y Scale.Scale Fit")) -> ()  [unwired: 2 in, 2 out]
      }
      event "Graph": Scale Range Change {
        n88 = event-data() -> ()  [unwired: 1 in, 8 out]
      }
      event "Graph": Autoscale Range Change {
        n89 = event-data() -> ("NewRange"=w111:T13)  [unwired: 1 in, 7 out]
        n90 = Unbundle By Name(w111) -> ()  [unwired: 2 out]
      }
      event "Graph": Plot Attribute Change {
        n91 = event-data() -> ()  [unwired: 1 in, 8 out]
      }
      event "DisconnectBtn": Value Change {
        n92 = event-data() -> ()  [unwired: 1 in, 6 out]
        n93 = stacked-sequence {
          tunnel: w114 -> [_ _ _ _ _ w129]
          frame #0 {
            n94 = Wait (ms)(milliseconds to wait=u32 1000) -> ()  [unwired: 1 out]
          }
          frame #1 {
            w117 = TRUE ("ConnectionStatus")
            n95 = property on="Blank Top" class="Bool (strict)"("Visible"=w117) -> ()  [unwired: 2 in, 2 out]
            n96 = property on="Blank Bottom" class="Bool (strict)"("Visible"=w117) -> ()  [unwired: 2 in, 2 out]
          }
          frame #2 {
            n97 = local write "error out"(errorcluster {"status"=TRUE, "code"=0, "source"=""} ("error out")) -> ()
            n98 = property on="Connect" class="Bool (strict)"("Visible"=TRUE) -> ()  [unwired: 2 in, 2 out]
            n99 = property on="DisconnectBtn" class="Bool (strict)"("Visible"=FALSE) -> ()  [unwired: 2 in, 2 out]
          }
          frame #3 {
            n100 = local read "VISA resource name"() -> (w123:refnum<visa-resource-name>)
            n101 = local write "DisconnectBtn"(FALSE ("DisconnectBtn")) -> ()
            n102 = VISA Close(VISA resource name=w123) -> (error out=w122:errorcluster)  [unwired: 1 in]
            n103 = call <vilib>:"Simple Error Handler.vi"("error in (no error)"=w122) -> ()  [unwired: 1 in, 8 out]
          }
          frame #4 {
            w124 = T10."Disabled" ("Disabled")
            n104 = property on="ServiceWin" class="Bool (strict)"("DisabledEnum"=w124) -> ()  [unwired: 2 in, 2 out]
            n105 = property on="CalibrB" class="Bool (strict)"("DisabledEnum"=w124) -> ()  [unwired: 2 in, 2 out]
            n106 = property on="DispB" class="Bool (strict)"("DisabledEnum"=w124) -> ()  [unwired: 2 in, 2 out]
            n107 = property on="Setngs485" class="Bool (strict)"("DisabledEnum"=w124) -> ()  [unwired: 2 in, 2 out]
            n108 = property on="Config" class="Bool (strict)"("DisabledEnum"=w124) -> ()  [unwired: 2 in, 2 out]
          }
          frame #5 {
            w127 = FALSE
            w126 = TRUE
            (unwired) T10."Enabled" ("Disabled")
            w130 = T10."Disabled" ("Disabled")
            n109 = VISA Close(VISA resource name=w129) -> ()  [unwired: 1 in, 1 out]
            n110 = property on="CalibrB" class="Bool (strict)"("DisabledEnum"=w130) -> ()  [unwired: 2 in, 2 out]
            n111 = property on="DispB" class="Bool (strict)"("DisabledEnum"=w130) -> ()  [unwired: 2 in, 2 out]
            n112 = property on="Setngs485" class="Bool (strict)"("DisabledEnum"=w130) -> ()  [unwired: 2 in, 2 out]
            n113 = property on="Config" class="Bool (strict)"("DisabledEnum"=w130) -> ()  [unwired: 2 in, 2 out]
            n114 = property on="Blank Top" class="Bool (strict)"("Visible"=w126) -> ()  [unwired: 2 in, 2 out]
            n115 = property on="Blank Bottom" class="Bool (strict)"("Visible"=w126) -> ()  [unwired: 2 in, 2 out]
            n116 = property on="Connect" class="Bool (strict)"("Visible"=w126) -> ()  [unwired: 2 in, 2 out]
            n117 = local write "Tab Control"(T2."Settings" ("Tab Control")) -> ()
            n118 = local write "Setngs485"(TRUE ("CalibrB")) -> ()
            n119 = property on="DisconnectBtn" class="Bool (strict)"("Visible"=w127) -> ()  [unwired: 2 in, 2 out]
            n120 = local write "CalibrB"(w127) -> ()
            n121 = local write "Config"(w127) -> ()
            n122 = local write "DispB"(w127) -> ()
          }
        }
        n123 = local write "ConnectionFlag"(FALSE ("ConnectionFlag")) -> ()
      }
      event "SavePointCal 2": Value Change {
        n124 = event-data() -> ()  [unwired: 1 in, 6 out]
        n125 = disable-structure shown="Disabled" {
          frame Disabled {
            n126 = stacked-sequence {
              frame #0 {
                (unwired) FALSE
              }
              frame #1 {
                n127 = property on="CalPointN" class="Ring (strict)"("DisabledEnum"=T10."Enabled" ("Disabled")) -> ()  [unwired: 2 in, 2 out]
                n128 = property on="SavePointCal 2" class="Bool"("DisabledEnum"=T10."Disabled" ("Disabled")) -> ()  [unwired: 2 in, 2 out]
              }
            }
          }
          frame Enabled {
          }
        }
        n129 = Equal?(x="CalPointN", y=u16 0) -> (x = y?=w134:bool)
        n130 = Select(t=enum16{"Temperature", "Pressure"}."Temperature" ("Mode 2"), s=w134, f=enum16{"Temperature", "Pressure"}."Pressure" ("Mode 2")) -> (s? t:f=w131:enum16{"Temperature", "Pressure"})
        n131 = call "Calibration.vi"("Enable"=w140, "New value"="CalibValue", "error in"=w137, "Mode"=w131, "Cluster"=w141, "VISA Refnum in"=w142) -> ("error out"=w139:errorcluster)  [unwired: 3 in, 2 out]
      }
      event "modeChange": Value Change {
        n132 = event-data() -> ()  [unwired: 1 in, 6 out]
        n133 = case shown="2, Default" "Mode" {
          selector: "Mode" -> [_ w153]
          tunnel: [w152 w153] -> w148
          frame 2, Default {
            n134 = call "SubVi.vi"() -> ("Mode"=w152:i32)  [unwired: 11 in]
          }
          frame 1 {
          }
        }
        n135 = call "ModeSelect.vi"("Mode in"=w148) -> ("Strings And Values []"=w150:T12, "Mode out"=→"Режим работы":u16)  [unwired: 9 in]
        n136 = Equal?(x=w148, y=2) -> (x = y?=w146:bool)
        n137 = property on="CalPointN" class="Ring (strict)"("StringsAndValues[]"=w150) -> ()  [unwired: 2 in, 2 out]
        n138 = property on="ServiceWin" class="Bool (strict)"("Visible"=w146) -> ()  [unwired: 2 in, 2 out]
        n139 = local write "Mode"(w148) -> ()
      }
      event "showDestiny": Value Change {
        n140 = event-data() -> ("NewVal"=w155:bool)  [unwired: 1 in, 5 out]
        n141 = property on="Graph" class="WFChart (strict)"("Active Plot"=u32 0, "Plot.Visible?"=w155) -> ()  [unwired: 2 in, 2 out]
      }
      event "showPressure": Value Change {
        n142 = event-data() -> ("NewVal"=w158:bool)  [unwired: 1 in, 5 out]
        n143 = property on="Graph" class="WFChart (strict)"("Active Plot"=u32 1, "Plot.Visible?"=w158) -> ()  [unwired: 2 in, 2 out]
      }
      event "showTemp": Value Change {
        n144 = event-data() -> ("NewVal"=w161:bool)  [unwired: 1 in, 5 out]
        n145 = property on="Graph" class="WFChart (strict)"("Active Plot"=u32 2, "Plot.Visible?"=w161) -> ()  [unwired: 2 in, 2 out]
      }
      event "showReducedPressure": Value Change {
        n146 = event-data() -> ("NewVal"=w164:bool)  [unwired: 1 in, 5 out]
        n147 = property on="Graph" class="WFChart (strict)"("Active Plot"=u32 3, "Plot.Visible?"=w164) -> ()  [unwired: 2 in, 2 out]
      }
      event "ReadCalData": Value Change {
        # "Загрузка графика АЦП - Концентрация"
        n148 = event-data() -> ()  [unwired: 1 in, 6 out]
        n149 = call "LoadGasCalibr.vi"("Enable"=w168, "Read"="ReadCalData", "error in (no error)"=w166, "Cluster"=w171, "VISA Refnum in"=w173) -> ("error out"=w167:errorcluster, "Array Graph"=→"XY graph 2":cluster{u16[], u16[]}[], "Array INT"=→"Array INT":i32[][])  [unwired: 4 in]
      }
      event "Setngs485": Value Change {
        w176 = T2."Settings" ("Tab Control")
        n150 = event-data() -> ()  [unwired: 1 in, 6 out]
        n151 = call "BlankArray.vi"() -> ("Array"=w179:bool[])  [unwired: 11 in]
        n152 = Replace Array Subset(array=w179, new element=TRUE ("SettingsB"), index=w176) -> (w180:bool[])
        n153 = local write "Tab Control"(w176) -> ()
        n154 = Index Array(array=w180, index #1=0 ("index")) -> (element #1=w183:bool, element #2=w182:bool, element #3=w177:bool, element #4=w178:bool, element #5=w175:bool)  [unwired: 4 in]
        n155 = local write "ServiceWin"(w175) -> ()
        n156 = local write "Setngs485"(w183) -> ()
        n157 = local write "CalibrB"(w182) -> ()
        n158 = local write "DispB"(w177) -> ()
        n159 = local write "Config"(w178) -> ()
      }
      event "Config": Value Change {
        w187 = T2."Config" ("Tab Control")
        n160 = event-data() -> ()  [unwired: 1 in, 6 out]
        n161 = call "BlankArray.vi"() -> ("Array"=w190:bool[])  [unwired: 11 in]
        n162 = Replace Array Subset(array=w190, new element=TRUE ("SettingsB"), index=w187) -> (w191:bool[])
        n163 = Index Array(array=w191, index #1=0 ("index")) -> (element #1=w194:bool, element #2=w193:bool, element #3=w189:bool, element #4=w188:bool, element #5=w186:bool)  [unwired: 4 in]
        n164 = local write "Tab Control"(w187) -> ()
        n165 = local write "ServiceWin"(w186) -> ()
        n166 = local write "Setngs485"(w194) -> ()
        n167 = local write "CalibrB"(w193) -> ()
        n168 = local write "Config"(w188) -> ()
        n169 = local write "DispB"(w189) -> ()
      }
      event "CalibrB": Value Change {
        w198 = T2."Calibration" ("Tab Control")
        n170 = event-data() -> ()  [unwired: 1 in, 6 out]
        n171 = call "BlankArray.vi"() -> ("Array"=w201:bool[])  [unwired: 11 in]
        n172 = local write "Tab Control"(w198) -> ()
        n173 = Replace Array Subset(array=w201, new element=TRUE ("SettingsB"), index=w198) -> (w202:bool[])
        n174 = Index Array(array=w202, index #1=0 ("index")) -> (element #1=w205:bool, element #2=w204:bool, element #3=w199:bool, element #4=w200:bool, element #5=w197:bool)  [unwired: 4 in]
        n175 = local write "Setngs485"(w205) -> ()
        n176 = local write "CalibrB"(w204) -> ()
        n177 = local write "Config"(w200) -> ()
        n178 = local write "DispB"(w199) -> ()
        n179 = local write "ServiceWin"(w197) -> ()
      }
      event "DispB": Value Change {
        w209 = T2."Display" ("Tab Control")
        n180 = event-data() -> ()  [unwired: 1 in, 6 out]
        n181 = local write "Tab Control"(w209) -> ()
        n182 = call "BlankArray.vi"() -> ("Array"=w212:bool[])  [unwired: 11 in]
        n183 = Replace Array Subset(array=w212, new element=TRUE ("SettingsB"), index=w209) -> (w213:bool[])
        n184 = Index Array(array=w213, index #1=0 ("index")) -> (element #1=w216:bool, element #2=w215:bool, element #3=w210:bool, element #4=w211:bool, element #5=w208:bool)  [unwired: 4 in]
        n185 = local write "Setngs485"(w216) -> ()
        n186 = local write "CalibrB"(w215) -> ()
        n187 = local write "DispB"(w210) -> ()
        n188 = local write "Config"(w211) -> ()
        n189 = local write "ServiceWin"(w208) -> ()
      }
      event "ServiceWin": Value Change {
        w221 = T2."Service" ("Tab Control")
        n190 = event-data() -> ()  [unwired: 1 in, 6 out]
        n191 = call "BlankArray.vi"() -> ("Array"=w223:bool[])  [unwired: 11 in]
        n192 = local write "Tab Control"(w221) -> ()
        n193 = Replace Array Subset(array=w223, new element=TRUE ("SettingsB"), index=w221) -> (w224:bool[])
        n194 = Index Array(array=w224, index #1=0 ("index")) -> (element #1=w227:bool, element #2=w226:bool, element #3=w219:bool, element #4=w222:bool, element #5=w220:bool)  [unwired: 4 in]
        n195 = local write "Setngs485"(w227) -> ()
        n196 = local write "CalibrB"(w226) -> ()
        n197 = local write "Config"(w222) -> ()
        n198 = local write "DispB"(w219) -> ()
        n199 = local write "ServiceWin"(w220) -> ()
      }
      event "Выкл": Value Change {
        n200 = event-data() -> ()  [unwired: 1 in, 6 out]
        n201 = Boolean To (0,1)(Boolean="HeaterBreakerSet") -> (0, 1=w232:i16)
        n202 = call "MB Write.vim"("VISA Refnum in"=w236, "Command"=u16 297 ("Holding Register"), "Data"=w232, "Cluster"=w234, "error in"=w229, "Enable"=w231) -> ("error out"=w230:errorcluster)  [unwired: 7 in, 2 out]
      }
      event "MagnetWrite": Value Change {
        n203 = event-data() -> ()  [unwired: 1 in, 6 out]
        n204 = Boolean To (0,1)(Boolean="MagnetSP") -> (0, 1=w241:i16)
        n205 = call "MB Write.vim"("VISA Refnum in"=w244, "Command"=u16 216 ("Holding Register"), "Data"=w241, "Cluster"=w242, "error in"=w237, "Enable"=w239) -> ("error out"=w238:errorcluster)  [unwired: 7 in, 2 out]
      }
      event "Заводские\nнастройки": Value Change {
        n206 = event-data() -> ()  [unwired: 1 in, 6 out]
        n207 = call "DialogBox.vi"("Caption.Text"="Вернуть к заводским\nнастройкам?" ("String")) -> ("Output"=w249:bool)  [unwired: 10 in]
        n208 = case shown="True" w249 {
          tunnel: w251 -> [_ w258]
          tunnel: w250 -> [_ w255]
          tunnel: w247 -> [_ w254]
          tunnel: [w252 w253] -> w246
          tunnel: w245 -> [w252 _]
          frame False {
          }
          frame True {
            n209 = call "MB Write.vim"("VISA Refnum in"=w258, "Command"=u16 48 ("Holding Register"), "Data"=u16 0, "Cluster"=w255, "Enable"=w254) -> ("error out"=w253:errorcluster)  [unwired: 8 in, 2 out]
          }
        }
      }
      event "Dirt Calibr": Value Change {
        n210 = event-data() -> ()  [unwired: 1 in, 6 out]
        n211 = call "MB Write.vim"("VISA Refnum in"=w265, "Command"=u16 99 ("Holding Register"), "Data"=u16 0, "Cluster"=w262, "error in"=w259, "Enable"=w261) -> ("error out"=w260:errorcluster)  [unwired: 7 in, 2 out]
      }
      event "Перезагрузка": Value Change {
        n212 = event-data() -> ()  [unwired: 1 in, 6 out]
        n213 = call "DialogBox.vi"("Caption.Text"="Перезагрузить\nдетектор?") -> ("Output"=w270:bool)  [unwired: 10 in]
        n214 = case shown="True" w270 {
          tunnel: w272 -> [_ w281]
          tunnel: w271 -> [_ w278]
          tunnel: w268 -> [_ w276]
          tunnel: [w273 w275] -> w267
          tunnel: w266 -> [w273 w274]
          frame False {
          }
          frame True {
            n215 = Tick Count (ms)() -> (millisecond timer value=w277:u32)
            n216 = call "MB Write.vim"("VISA Refnum in"=w281, "Command"=u16 594 ("Holding Register"), "Data"=u16 0, "Cluster"=w278, "error in"=w274, "Enable"=w276) -> ("error out"=w275:errorcluster)  [unwired: 7 in, 2 out]
            n217 = while {
              tunnel: w277 -> [w287]
              stop <- w283 stop-if-true
              n218 = Tick Count (ms)() -> (millisecond timer value=w288:u32)
              n219 = Subtract(x=w288, y=w287) -> (x-y=w286:u32)
              n220 = Multiply(x=0.001, y=w286) -> (x*y=w282:dbl)
              "ResetTi" <- w282
              n221 = Less?(x=u32 11 ("milliseconds to wait"), y=w282) -> (x < y?=w283:bool)
            }
          }
        }
      }
      event "Setfirm": Value Change {
        n222 = event-data() -> ()  [unwired: 1 in, 6 out]
        n223 = call "PresetServiceData.vi"("Data"="Firmware", "Enable"=w291, "Command"=u16 591, "error in"=w289, "Cluster in"=w294, "VISA Refnum in"=w295) -> ("error out"=w290:errorcluster)  [unwired: 3 in, 2 out]
      }
      event "SaveTLog?": Value Change {
        n224 = event-data() -> ()  [unwired: 1 in, 6 out]
        n225 = case shown="True" "SaveTLog?" {
          selector: "SaveTLog?" -> [w299 _]
          tunnel: [w299 w301] -> w298
          frame False {
          }
          frame True {
            n226 = call "SaveTempCalibrLog.vi"() -> ("selected path"=→"File Path":path, "Boolean"=w301:bool)  [unwired: 10 in]
          }
        }
        n227 = local write "SaveTLog?"(w298) -> ()
      }
      event "SetSerialN": Value Change {
        n228 = event-data() -> ()  [unwired: 1 in, 6 out]
        n229 = call "PresetServiceData.vi"("Data"="SerialNumber", "Enable"=w304, "Command"=u16 590, "error in"=w302, "Cluster in"=w306, "VISA Refnum in"=w307) -> ("error out"=w303:errorcluster)  [unwired: 3 in, 2 out]
      }
      event "ClearTGraph": Value Change {
        n230 = event-data() -> ()  [unwired: 1 in, 6 out]
        n231 = property on="Temp/Press" class="WFChart (strict)"("History Data"=T15 []) -> ()  [unwired: 2 in, 2 out]
      }
      event "FitRawGraph": Value Change {
        n232 = event-data() -> ()  [unwired: 1 in, 6 out]
        n233 = disable-structure shown="Disabled" {
          frame Disabled {
            n234 = local read "Sensor"() -> (w313:T6)
            n235 = case shown="\"Radio Selection 6\"" {
              selector: _ -> [_ _ _ _ _ _]
              tunnel: w313 -> [w322 w324 w326 w328 w330 w332]
              tunnel: [w321 w323 w325 w327 w329 w331] -> w312
              frame "Radio Selection 1", Default {
                n236 = Unbundle(w322) -> ("Numeric"=w321:dbl)  [unwired: 4 out]
              }
              frame "Radio Selection 2" {
                n237 = Unbundle(w324) -> ("Numeric"=w323:dbl)  [unwired: 4 out]
              }
              frame "Radio Selection 3" {
                n238 = Unbundle(w326) -> ("Numeric"=w325:dbl)  [unwired: 4 out]
              }
              frame "Radio Selection 4" {
                n239 = Unbundle(w328) -> ("Numeric"=w327:dbl)  [unwired: 4 out]
              }
              frame "Radio Selection 5" {
                n240 = Unbundle(w330) -> ("Numeric"=w329:dbl)  [unwired: 4 out]
              }
              frame "Radio Selection 6" {
                n241 = Unbundle(w332) -> ("Numeric"=w331:dbl)  [unwired: 4 out]
              }
            }
            n242 = Build Array(w312) -> (w320:dbl[])
            n243 = Array Max & Min(array=w320) -> (max value=w315:dbl, min value=w314:dbl)  [unwired: 2 out]
            n244 = Multiply(x=w314, y=0.98) -> (x*y=w319:dbl)
            n245 = Multiply(x=w315, y=1.01) -> (x*y=w318:dbl)
            n246 = property on="Sensor" class="WFChart (strict)"("YScale.Maximum"=w318, "YScale.Minimum"=w319) -> ()  [unwired: 2 in, 2 out]
          }
          frame Enabled {
          }
        }
      }
      event "Visible1": Value Change {
        w338 = u32 2 ("Active Plot")
        n247 = event-data() -> ()  [unwired: 1 in, 6 out]
        n248 = Not(x="Visible1") -> (.not. x?=w337:bool)
        n249 = Replace Array Subset(array=w335, new element="Visible1", index=w338) -> (w334:bool[])
        n250 = property on="Sensor" class="WFChart (strict)"("Active Plot"=w338, "Plot.Visible?"=w337) -> ()  [unwired: 2 in, 2 out]
        n251 = local write "visibleArray"(w334) -> ()
      }
      event "Visible2": Value Change {
        w344 = u32 0 ("Active Plot")
        n252 = event-data() -> ()  [unwired: 1 in, 6 out]
        n253 = Not(x="Visible2") -> (.not. x?=w343:bool)
        n254 = Replace Array Subset(array=w342, new element="Visible2", index=w344) -> (w341:bool[])
        n255 = property on="Sensor" class="WFChart (strict)"("Active Plot"=w344, "Plot.Visible?"=w343) -> ()  [unwired: 2 in, 2 out]
        n256 = local write "visibleArray"(w341) -> ()
      }
      event "Visible3": Value Change {
        w350 = u32 1 ("Active Plot")
        n257 = event-data() -> ()  [unwired: 1 in, 6 out]
        n258 = Not(x="Visible3") -> (.not. x?=w349:bool)
        n259 = Replace Array Subset(array=w348, new element="Visible3", index=w350) -> (w347:bool[])
        n260 = property on="Sensor" class="WFChart (strict)"("Active Plot"=w350, "Plot.Visible?"=w349) -> ()  [unwired: 2 in, 2 out]
        n261 = local write "visibleArray"(w347) -> ()
      }
      event "Visible4": Value Change {
        w356 = u32 3 ("Active Plot")
        n262 = event-data() -> ()  [unwired: 1 in, 6 out]
        n263 = Not(x="Visible4") -> (.not. x?=w355:bool)
        n264 = Replace Array Subset(array=w354, new element="Visible4", index=w356) -> (w353:bool[])
        n265 = property on="Sensor" class="WFChart (strict)"("Active Plot"=w356, "Plot.Visible?"=w355) -> ()  [unwired: 2 in, 2 out]
        n266 = local write "visibleArray"(w353) -> ()
      }
      event "Visible5": Value Change {
        w362 = u32 4 ("Active Plot")
        n267 = event-data() -> ()  [unwired: 1 in, 6 out]
        n268 = Not(x="Visible5") -> (.not. x?=w361:bool)
        n269 = Replace Array Subset(array=w360, new element="Visible5", index=w362) -> (w359:bool[])
        n270 = property on="Sensor" class="WFChart (strict)"("Active Plot"=w362, "Plot.Visible?"=w361) -> ()  [unwired: 2 in, 2 out]
        n271 = local write "visibleArray"(w359) -> ()
      }
      event "ClearRAWGraph": Value Change {
        n272 = event-data() -> ()  [unwired: 1 in, 6 out]
        n273 = property on="Sensor" class="WFChart (strict)"("History Data"=T16 []) -> ()  [unwired: 2 in, 2 out]
      }
      event "ZeroShiftSetBtn": Value Change {
        n274 = event-data() -> ()  [unwired: 1 in, 6 out]
        n275 = call "MB Write.vim"("VISA Refnum in"=w369, "Command"=u16 88, "Data"="ZeroShiftSet", "Cluster"=w368, "error in"=w365, "Enable"=w367) -> ("error out"=w366:errorcluster)  [unwired: 7 in, 2 out]
      }
      event "heatUpLimW": Value Change {
        n276 = event-data() -> ()  [unwired: 1 in, 6 out]
        n277 = call "MB Write.vim"("VISA Refnum in"=w377, "Command"=u16 596, "Data"="heatUpLimSP", "Cluster"=w376, "error in"=w372, "Enable"=w374) -> ("error out"=w373:errorcluster)  [unwired: 7 in, 2 out]
      }
      event "heatLowLimW": Value Change {
        n278 = event-data() -> ()  [unwired: 1 in, 6 out]
        n279 = call "MB Write.vim"("VISA Refnum in"=w384, "Command"=u16 595, "Data"="heatLowLimSP", "Cluster"=w383, "error in"=w379, "Enable"=w381) -> ("error out"=w380:errorcluster)  [unwired: 7 in, 2 out]
      }
      event "WirenSetMode": Value Change {
        n280 = event-data() -> ()  [unwired: 1 in, 6 out]
        n281 = Boolean To (0,1)(Boolean="WirenSet") -> (0, 1=w390:i16)
        n282 = call "MB Write.vim"("VISA Refnum in"=w392, "Command"=u16 304, "Data"=w390, "Cluster"=w391, "error in"=w386, "Enable"=w388) -> ("error out"=w387:errorcluster)  [unwired: 7 in, 2 out]
      }
      event "IRSetBtn": Value Change {
        n283 = event-data() -> ()  [unwired: 1 in, 6 out]
        n284 = call "MB Write.vim"("VISA Refnum in"=w400, "Command"=u16 214, "Data"="IR Time", "Cluster"=w399, "error in"=w394, "Enable"=w396) -> ("error out"=w395:errorcluster)  [unwired: 7 in, 2 out]
      }
      event "TaskSet": Value Change {
        n285 = event-data() -> ()  [unwired: 1 in, 6 out]
        n286 = call "MB Write.vim"("VISA Refnum in"=w407, "Command"=u16 210, "Data"="TaskTime", "Cluster"=w406, "error in"=w401, "Enable"=w403) -> ("error out"=w402:errorcluster)  [unwired: 7 in, 2 out]
      }
      event "SetGain": Value Change {
        n287 = event-data() -> ()  [unwired: 1 in, 6 out]
        n288 = Boolean To (0,1)(Boolean="OK Button") -> (0, 1=w411:i16)
        n289 = call "MB Write.vim"("VISA Refnum in"=w415, "Command"=u16 299, "Data"=w411, "Cluster"=w414, "error in"=w408, "Enable"=w410) -> ("error out"=w409:errorcluster)  [unwired: 7 in, 2 out]
      }
      event "BlockErrorSet": Value Change {
        n290 = event-data() -> ()  [unwired: 1 in, 6 out]
        n291 = Build Array("Err 0", "Err 1", "Err 2", "Err 3", "Err 4", "Err 5", "Err 6", "Err 7") -> (w420:bool[])
        n292 = Boolean Array To Number(Boolean array=w420) -> (number=w419:u32)
        n293 = call "MB Write.vim"("VISA Refnum in"=w430, "Command"=u16 50 ("Holding Register"), "Data"=w419, "Cluster"=w431, "error in"=w416, "Enable"=w418) -> ("error out"=w417:errorcluster)  [unwired: 7 in, 2 out]
      }
      event "getCorner": Value Change {
        n294 = event-data() -> ()  [unwired: 1 in, 6 out]
        n295 = case shown="True" w434 {
          tunnel: w440 -> [_ w449]
          tunnel: w439 -> [_ w448]
          tunnel: [u16[] [] ("Holding Registers") w445] -> w438
          tunnel: [w441 w444] -> w433
          tunnel: w432 -> [w441 w443]
          frame False {
          }
          frame True {
            n296 = call <vilib>:"MB Serial Master Query Read Holding Registers (poly).vi"("VISA resource name"=w448, "Starting Address"=u16 522, "Quantity"=u16 3 ("Starting Address"), "error in"=w443, "Serial Parameters"=w449) -> ("Holding Registers"=w445:u16[], "error out"=w444:errorcluster)  [unwired: 11 in, 2 out]
          }
        }
        n297 = Index Array(array=w438) -> (element #1=→"cornerGas":u16, element #2=→"cornerRef":u16, element #3=→"spanZ":u16)  [unwired: 3 in]
      }
      event "ContaminSet": Value Change {
        n298 = event-data() -> ()  [unwired: 1 in, 6 out]
        n299 = call "MB Write.vim"("VISA Refnum in"=w455, "Command"=u16 78 ("Holding Register"), "Data"="ContaminantSetPoint", "Cluster"=w456, "error in"=w450, "Enable"=w452) -> ("error out"=w451:errorcluster)  [unwired: 7 in, 2 out]
      }
      event "stablePirSP_Set": Value Change {
        n300 = event-data() -> ()  [unwired: 1 in, 6 out]
        n301 = call "MB Write.vim"("VISA Refnum in"=w462, "Command"=u16 225 ("Holding Register"), "Data"="stablePirSP", "Cluster"=w463, "error in"=w457, "Enable"=w459) -> ("error out"=w458:errorcluster)  [unwired: 7 in, 2 out]
      }
      event "refNoiseSP_set": Value Change {
        n302 = event-data() -> ()  [unwired: 1 in, 6 out]
        n303 = call "MB Write.vim"("VISA Refnum in"=w469, "Command"=u16 226 ("Holding Register"), "Data"="refNoiseSP", "Cluster"=w470, "error in"=w464, "Enable"=w466) -> ("error out"=w465:errorcluster)  [unwired: 7 in, 2 out]
      }
      event "gasNoise_set": Value Change {
        n304 = event-data() -> ()  [unwired: 1 in, 6 out]
        n305 = call "MB Write.vim"("VISA Refnum in"=w476, "Command"=u16 227 ("Holding Register"), "Data"="gasNoiseSP", "Cluster"=w477, "error in"=w471, "Enable"=w473) -> ("error out"=w472:errorcluster)  [unwired: 7 in, 2 out]
      }
      event "thermoGradientSP_Set": Value Change {
        n306 = event-data() -> ()  [unwired: 1 in, 6 out]
        n307 = call "MB Write.vim"("VISA Refnum in"=w483, "Command"=u16 228 ("Holding Register"), "Data"="thermoGradientSP", "Cluster"=w484, "error in"=w478, "Enable"=w480) -> ("error out"=w479:errorcluster)  [unwired: 7 in, 2 out]
      }
      event "Update": Value Change {
        w486 = T14 2 items=["Canonical Names Only"=0, "Aliases Only"=2, "Include Matching Aliases"=3, "Include All Aliases"=4] ("Search Mode")
        n308 = event-data() -> ()  [unwired: 1 in, 6 out]
        n309 = VISA Find Resource(10:w486) -> (2:w487:u32, 3:w488:string[])  [unwired: 2 in, 1 out]
        "find list" <- w488
        n310 = call "GetDeviceName.vi"("PortQuantity"=w487, "Input"=w488) -> ("Output"=w489:string[])  [unwired: 9 in]
        n311 = property on="Порт" class="Ring (strict)"("Strings []"=w489) -> ()  [unwired: 2 in, 2 out]
      }
      event "Connect": Value Change {
        n312 = event-data() -> ()  [unwired: 1 in, 6 out]
        n313 = call <vilib>:"Clear Errors.vi"("error in (no error)"=w491) -> ("error out"=w490:errorcluster)  [unwired: 5 in, 1 out]
        n314 = stacked-sequence {
          seq-local: [_ w499 _] -> [_ _ w515]
          tunnel: "Connect" -> [_ _ _]
          tunnel: [_ _ w515] -> w492
          tunnel: w490 -> [_ w497 _]
          frame #0 {
            n315 = local write "CC1"(TRUE ("CC1")) -> ()
            n316 = property on="Connect" class="Bool (strict)"("DisabledEnum"=T10."Disabled" ("Disabled")) -> ()  [unwired: 2 in, 2 out]
            n317 = local write "Lost"(i16 0 ("Lost")) -> ()
          }
          frame #1 {
            n318 = local read "find list"() -> (w508:string[])
            n319 = call "Get Connection to Detector.vi"("BAUD"="BAUD", "Mode"="Mode", "error in (no error)"=w497, "Порт"="Порт", "find list"=w508, "Адрес датчика"="Адрес датчика") -> ("error out"=w498:errorcluster, "SN"=→"Serial":u16, "FW"=→"FirmW":u16, "VISA Refnum out"=w504:refnum<visa-resource-name>, "p_atm"=w507:sgl, "Cluster"=w503:T1)
            "VISA resource name" <- w504
            "Cluster" <- w503
            n320 = local write "Плотность"(w507) -> ()
            n321 = property on="Pressure units" class="Enum (strict)"() -> ("Strings []"=w506:string[])  [unwired: 2 in, 2 out]
            n322 = call "Read Register.vi"("Refnum in"=w504, "startReg"=u16 4 ("Command"), "Mode"=w503, "error in (no error)"=w498, "Enable"=TRUE) -> ("Numeric"=w500:u16, "error out"=w499:errorcluster)  [unwired: 6 in, 3 out]
            "error out" <- w499
            n323 = Index Array(array=w506, index=w500) -> (element=→"Pressure meas" →"Pressure meas 2":string)
            n324 = local write "Pressure units"(w500) -> ()
            "Адрес" <- "Адрес датчика"
          }
          frame #2 {
            n325 = Unbundle By Name(w515) -> ("status"=w517:bool)
            n326 = local read "Temp units"() -> (w519:dbl)
            n327 = Multiply(x=w519, y=10.0) -> (x*y=w520:dbl)
            n328 = Not(x=w517) -> (.not. x?=→"ConnectionFlag":bool)
            n329 = case shown="0, Default" w520 {
              tunnel: ["°С" ("Temp meas") "F" ("Temp meas") "K" ("Temp meas")] -> w521
              frame 0, Default {
              }
              frame 320 {
              }
              frame 2735 {
              }
            }
            "Temp meas" <- w521
            n330 = property on="Connect" class="Bool (strict)"("DisabledEnum"=T10."Enabled" ("Disabled")) -> ()  [unwired: 2 in, 2 out]
            n331 = case shown="False" FALSE {
              frame False {
                n332 = stacked-sequence {
                  frame #0 {
                    n333 = local write "Connect"(FALSE ("Connect")) -> ()
                    n334 = property on="ConnectionStatus" class="Bool (strict)"("Visible"=TRUE) -> ()  [unwired: 2 in, 2 out]
                  }
                  frame #1 {
                    n335 = property on="DisconnectBtn" class="Bool (strict)"("Visible"=TRUE) -> ()  [unwired: 2 in, 2 out]
                    n336 = property on="Connect" class="Bool (strict)"("DisabledEnum"=T10."Enabled" ("Disabled")) -> ()  [unwired: 2 in, 2 out]
                    n337 = property on="Connect" class="Bool (strict)"("Visible"=FALSE) -> ()  [unwired: 2 in, 2 out]
                  }
                  frame #2 {
                    w532 = FALSE ("Connect")
                    n338 = property on="Blank Bottom" class="Bool (strict)"("Visible"=w532) -> ()  [unwired: 2 in, 2 out]
                    n339 = property on="Blank Top" class="Bool (strict)"("Visible"=w532) -> ()  [unwired: 2 in, 2 out]
                  }
                  frame #3 {
                    w533 = T10."Enabled" ("Disabled")
                    n340 = property on="CalibrB" class="Bool (strict)"("DisabledEnum"=w533) -> ()  [unwired: 2 in, 2 out]
                    n341 = property on="DispB" class="Bool (strict)"("DisabledEnum"=w533) -> ()  [unwired: 2 in, 2 out]
                    n342 = property on="Setngs485" class="Bool (strict)"("DisabledEnum"=w533) -> ()  [unwired: 2 in, 2 out]
                    n343 = property on="Config" class="Bool (strict)"("DisabledEnum"=w533) -> ()  [unwired: 2 in, 2 out]
                    n344 = property on="ServiceWin" class="Bool (strict)"("DisabledEnum"=w533) -> ()  [unwired: 2 in, 2 out]
                  }
                }
              }
              frame True {
                (unwired) T10."Enabled" ("Disabled")
                w534 = FALSE
                n345 = local write "Connect"(FALSE) -> ()
                n346 = local write "CC2"(w534) -> ()
                n347 = local write "CC3"(w534) -> ()
                n348 = local write "CC1"(w534) -> ()
              }
            }
          }
        }
      }
      event "Create Backup": Value Change {
        n349 = event-data() -> ()  [unwired: 1 in, 6 out]
        n350 = call "Save BackUp.vi"("Refnum in"=w537, "Mode"=w538, "error in (no error)"=w536, "Enable"=w540) -> ("error out"=w539:errorcluster)  [unwired: 9 in, 2 out]
      }
      event "Load Backup": Value Change {
        n351 = event-data() -> ()  [unwired: 1 in, 6 out]
        n352 = call "Load settings from backup.vi"("Enable"=w545, "error in (no error)"=w541, "Cluster in"=w543, "VISA Refnum in"=w544) -> ("error out"=w542:errorcluster)  [unwired: 5 in, 2 out]
      }
      event "LowSignalBtnSet": Value Change {
        n353 = event-data() -> ()  [unwired: 1 in, 6 out]
        n354 = call "MB Write.vim"("VISA Refnum in"=w550, "Command"=u16 12 ("Holding Register"), "Data"="DirtKoefRSet 2", "Cluster"=w551, "Enable"=w547) -> ("error out"=w546:errorcluster)  [unwired: 8 in, 2 out]
      }
      event "Change Destiny": Value Change {
        w561 = u32 50 ("milliseconds to wait")
        w558 = u16 62
        # "Значение плотности - float\n1. разложить на 2 инт\n2. записать.\n3. сохранить настройку\n4. считать плотность из датчика"
        n355 = event-data() -> ()  [unwired: 1 in, 6 out]
        n356 = call "MB Write.vim"("VISA Refnum in"=w569, "Command"=w558, "Data"="NewDestiny", "Cluster"=w568, "Enable"=w556) -> ("VISA out"=w567:refnum<visa-resource-name>, "Cluster Out"=w564:T1, "error out"=w563:errorcluster)  [unwired: 8 in]
        n357 = call "Stall Data Flow.vim"("value in"=w567, "milliseconds to wait"=w561) -> ("value out"=w565:refnum<visa-resource-name>)  [unwired: 1 out]
        n358 = call "Save Settings.vi"("Enable"=w556, "error in"=w563, "Cluster"=w564, "VISA Refnum in"=w565) -> ("error out"=w557:errorcluster, "Cluster Out"=w559:T18, "VISA out"=w562:refnum<visa-resource-name>)  [unwired: 5 in]
        n359 = call "Stall Data Flow.vim"("value in"=w562, "milliseconds to wait"=w561) -> ("value out"=w560:refnum<visa-resource-name>)  [unwired: 1 out]
        n360 = call "Read Register (float).vi"("Refnum in"=w560, "startReg"=w558, "Mode"=w559, "WordCount"=u16 2, "Register type"=enum16{"Input", "Holding"}."Holding", "error in (no error)"=w557, "Enable"=w556) -> ("first element"=→"Плотность":sgl, "error out"=w552:errorcluster)  [unwired: 4 in, 3 out]
      }
      event "ChangePressureUnits": Value Change {
        w583 = u32 50 ("milliseconds to wait")
        w576 = u16 4
        # "Значение плотности - float\n1. разложить на 2 инт\n2. записать.\n3. сохранить настройку\n4. считать плотность из датчика"
        n361 = event-data() -> ()  [unwired: 1 in, 6 out]
        n362 = To Unsigned Word Integer(number="Pressure units new") -> (unsigned 16bit integer=w581:u16)
        n363 = call "MB Write.vim"("VISA Refnum in"=w590, "Command"=w576, "Data"=w581, "Cluster"=w589, "Enable"=w574) -> ("VISA out"=w588:refnum<visa-resource-name>, "Cluster Out"=w586:T1, "error out"=w585:errorcluster)  [unwired: 8 in]
        n364 = call "Stall Data Flow.vim"("value in"=w588, "milliseconds to wait"=w583) -> ("value out"=w587:refnum<visa-resource-name>)  [unwired: 1 out]
        n365 = call "Save Settings.vi"("Enable"=w574, "error in"=w585, "Cluster"=w586, "VISA Refnum in"=w587) -> ("error out"=w577:errorcluster, "Cluster Out"=w579:T18, "VISA out"=w584:refnum<visa-resource-name>)  [unwired: 5 in]
        n366 = call "Stall Data Flow.vim"("value in"=w584, "milliseconds to wait"=w583) -> ("value out"=w580:refnum<visa-resource-name>)  [unwired: 1 out]
        n367 = property on="Pressure units" class="Enum (strict)"() -> ("Strings []"=w572:string[])  [unwired: 2 in, 2 out]
        n368 = call "Read Register.vi"("Refnum in"=w580, "startReg"=w576, "Quantity"=u16 1 ("WordCount"), "Mode"=w579, "Register type"=enum16{"Input", "Holding"}."Holding", "error in (no error)"=w577, "Enable"=w574) -> ("Numeric"=w571:u16, "error out"=w573:errorcluster)  [unwired: 4 in, 3 out]
        n369 = local write "Pressure units"(w571) -> ()
        n370 = Index Array(array=w572, index=w571) -> (element=w570:string)
        n371 = local write "Pressure meas"(w570) -> ()
        n372 = local write "Pressure meas 2"(w570) -> ()
      }
      event "ChangeTempUnits": Value Change {
        n373 = event-data() -> ()  [unwired: 1 in, 6 out]
        n374 = Multiply(x="Temp units new", y=10.0) -> (x*y=w595:dbl)
        n375 = local write "Temp units"("Temp units new") -> ()
        n376 = case shown="2735" w595 {
          tunnel: ["°С" ("Temp meas") "F" ("Temp meas") "K" ("Temp meas")] -> w592
          frame 0, Default {
          }
          frame 320 {
          }
          frame 2735 {
          }
        }
        n377 = local write "Temp meas"(w592) -> ()
      }
      event "VerificationBtnSet": Value Change {
        n378 = event-data() -> ()  [unwired: 1 in, 6 out]
        n379 = call "PresetServiceData.vi"("Data"="Year", "Enable"=w601, "Command"=u16 592, "Cluster in"=w602, "VISA Refnum in"=w603) -> ("error out"=w600:errorcluster, "Cluster Out"=w608:T18, "VISA resource name out"=w609:refnum<visa-resource-name>)  [unwired: 4 in]
        n380 = call "PresetServiceData.vi"("Data"="Month", "Enable"=w601, "Command"=u16 593, "error in"=w600, "Cluster in"=w608, "VISA Refnum in"=w609) -> ("error out"=w599:errorcluster)  [unwired: 3 in, 2 out]
      }
      event "ThermoTableBtnW": Value Change {
        n381 = event-data() -> ()  [unwired: 1 in, 6 out]
        n382 = call "UploadCalibrDataFromTXT.vi"("Enable"=w611, "Cluster in"=w613, "VISA Refnum in"=w614) -> ("error out"=w610:errorcluster, "transposed array"=w612:i64[][])  [unwired: 6 in]
        n383 = local write "Array INT Temp"(w612) -> ()
      }
      event "DirtKoefBtnW": Value Change {
        n384 = event-data() -> ()  [unwired: 1 in, 6 out]
        n385 = call "MB Write.vim"("VISA Refnum in"=w619, "Command"=u16 200 ("Holding Register"), "Data"="DirtKoefRSet", "Cluster"=w620, "Enable"=w616) -> ("error out"=w615:errorcluster)  [unwired: 8 in, 2 out]
      }
      event "ReadTermoData": Value Change {
        n386 = event-data() -> ()  [unwired: 1 in, 6 out]
        n387 = call "GetCalibrData.vi"("Mode"=w632, "Refnum in"=w633) -> ("error out"=w621:errorcluster, "INT"=w631:i32[][])  [unwired: 8 in]
        "Array INT Temp" <- w631
        n388 = Transpose 2D Array(2D array=w631) -> (transposed array=w630:i32[][])
        n389 = Index Array(array=w630, index (row) #1=0 ("index (row)"), index (row) #2=1 ("index (row)"), index (row) #3=2 ("index (row)")) -> (element #1=w625:i32[], element #2=w626:i32[], element #3=w624:i32[])  [unwired: 3 in]
        n390 = Bundle(w625, w626) -> (→"XY graph 3":cluster{i32[], i32[]})  [unwired: 1 in]
        n391 = Bundle(w625, w624) -> (→"XY graph 4":cluster{i32[], i32[]})  [unwired: 1 in]
      }
      event "SaveTermo": Value Change {
        n392 = event-data() -> ()  [unwired: 1 in, 6 out]
        n393 = local read "Array INT Temp"() -> (w639:i32[][])
        n394 = Transpose 2D Array(2D array=w639) -> (transposed array=w638:i32[][])
        n395 = Number To Decimal String(number=w638) -> (decimal integer string=w636:string[][])  [unwired: 1 in]
        n396 = call "SaveTempCalibrLog.vi"() -> ("selected path"=w634:path)  [unwired: 10 in, 1 out]
        n397 = call-poly <vilib>:"Write Delimited Spreadsheet.vi"("file path (dialog if empty)"=w634, "2D data"=w636, "append to file? (new file:F)"=TRUE) -> ()  [unwired: 11 in, 2 out]
      }
      event "SaveGasCalibr": Value Change {
        n398 = event-data() -> ()  [unwired: 1 in, 6 out]
        n399 = local read "Array INT"() -> (w644:i32[][])
        n400 = call "SaveTempCalibrLog.vi"() -> ("selected path"=w641:path)  [unwired: 10 in, 1 out]
        n401 = Number To Decimal String(number=w644) -> (decimal integer string=w642:string[][])  [unwired: 1 in]
        n402 = call-poly <vilib>:"Write Delimited Spreadsheet.vi"("file path (dialog if empty)"=w641, "2D data"=w642, "append to file? (new file:F)"=TRUE) -> ()  [unwired: 11 in, 2 out]
      }
      event "WriteCalibrData": Value Change {
        n403 = event-data() -> ()  [unwired: 1 in, 6 out]
        n404 = call "GasData.vi"("file path (dialog if empty)"="file path (dialog if empty)", "Cluster in"=w647, "VISA Refnum in"=w649) -> ("error out"=w645:errorcluster, "ArrayINT"=w646:i64[][])  [unwired: 7 in]
        n405 = local write "Array INT"(w646) -> ()
      }
      event "ChangeSlaveAdress": Value Change {
        w662 = u32 50 ("milliseconds to wait")
        w655 = u16 55 ("element")
        # "Смена адреса датчика"
        n406 = event-data() -> ()  [unwired: 1 in, 6 out]
        n407 = call "MB Write.vim"("VISA Refnum in"=w661, "Command"=w655, "Data"="NewSlave", "Cluster"=w660, "Enable"=w651) -> ("VISA out"=w667:refnum<visa-resource-name>, "Cluster Out"=w665:T1, "error out"=w664:errorcluster)  [unwired: 8 in]
        n408 = call "Stall Data Flow.vim"("value in"=w667, "milliseconds to wait"=w662) -> ("value out"=w666:refnum<visa-resource-name>)  [unwired: 1 out]
        n409 = call "Save Settings.vi"("Enable"=w651, "error in"=w664, "Cluster"=w665, "VISA Refnum in"=w666) -> ("error out"=w654:errorcluster, "Cluster Out"=w656:T18, "VISA out"=w663:refnum<visa-resource-name>)  [unwired: 5 in]
        n410 = call "Stall Data Flow.vim"("value in"=w663, "milliseconds to wait"=w662) -> ("value out"=w657:refnum<visa-resource-name>)  [unwired: 1 out]
        n411 = call "Read Register.vi"("Refnum in"=w657, "startReg"=w655, "Quantity"=u16 1 ("WordCount"), "Mode"=w656, "Register type"=enum16{"Input", "Holding"}."Holding", "error in (no error)"=w654, "Enable"=w651) -> ("Numeric"=w652:u16, "error out"=w653:errorcluster)  [unwired: 4 in, 3 out]
        n412 = local write "Адрес датчика"(w652) -> ()
        n413 = local write "Адрес"(w652) -> ()
        n414 = Bundle("Mode"=enum16{"RTU", "ASCII"}."RTU", "Numeric"=w652) -> (w668:T19)  [unwired: 1 in]
        n415 = local write "Cluster"(w668) -> ()
      }
      event "Tab Service": Value Change {
        n416 = event-data() -> ()  [unwired: 1 in, 6 out]
        n417 = case shown="\"Фильтр\"" "Tab Service" {
          tunnel: w675 -> [_ w681 w734]
          tunnel: w674 -> [_ w680 w735]
          tunnel: w672 -> [_ w678 w728]
          tunnel: [w676 w677 w727] -> w671
          tunnel: w670 -> [w676 _ _]
          frame "Графики", Default {
          }
          frame "Сервисные настройки" {
            n418 = call "GetConfig.vi"("Enable"=w678, "Cluster"=w681, "VISA Refnum in"=w680) -> ("error out"=w677:errorcluster, "output array"=w679:i32[])  [unwired: 7 in]
            n419 = stacked-sequence {
              tunnel: w679 -> [w689 w699 w706 w725]
              frame #0 {
                n420 = Index Array(array=w689, index #1=0 ("index")) -> (element #1=→"Год":i32, element #2=→"Месяц":i32, element #3=→"DirtChRead":i32, element #4=→"ZeroShifr":i32, element #5=w684:i32, element #6=→"LowLevelRead":i32, element #7=→"DirtKoefR":i32)  [unwired: 6 in]
                n421 = Number To Boolean Array(number=w684) -> (Boolean array=w693:bool[])
                n422 = Index Array(array=w693, index=0) -> (element=→"HeatRead":bool)
              }
              frame #1 {
                n423 = Index Array(array=w699, index #1=7 ("index")) -> (element #1=w698:i32, element #2=→"IR Time R":i32, element #3=→"TaskTimeRead":i32, element #4=→"heatUpLimRd_":i32, element #5=→"heatLowLimRd_":i32)  [unwired: 4 in]
                n424 = Number To Boolean Array(number=w698) -> (Boolean array=w702:bool[])
                n425 = Index Array(array=w702, index=0) -> (element=→"WirenMode_":bool)
              }
              frame #2 {
                n426 = Index Array(array=w706, index=12) -> (element=w704:i32)
                n427 = Number To Boolean Array(number=w704) -> (Boolean array=w707:bool[])
                n428 = Index Array(array=w707, index #1=0 ("index")) -> (element #1=w709:bool, element #2=w710:bool, element #3=w711:bool, element #4=w712:bool, element #5=w713:bool, element #6=w714:bool, element #7=w715:bool, element #8=w716:bool)  [unwired: 7 in]
                n429 = local write "Err 0"(w709) -> ()
                n430 = local write "Err 1"(w710) -> ()
                n431 = local write "Err 2"(w711) -> ()
                n432 = local write "Err 3"(w712) -> ()
                n433 = local write "Err 4"(w713) -> ()
                n434 = local write "Err 5"(w714) -> ()
                n435 = local write "Err 6"(w715) -> ()
                n436 = local write "Err 7"(w716) -> ()
              }
              frame #3 {
                n437 = Index Array(array=w725, index #1=13 ("index")) -> (element #1=w722:i32, element #2=w717:i32)  [unwired: 1 in]
                n438 = Number To Boolean Array(number=w722) -> (Boolean array=w723:bool[])
                n439 = Number To Boolean Array(number=w717) -> (Boolean array=w719:bool[])
                n440 = Index Array(array=w723, index=0) -> (element=→"gainLED":bool)
                n441 = Index Array(array=w719, index=0) -> (element=→"MagnetRead":bool)
              }
            }
          }
          frame "Фильтр" {
            n442 = call "Read Register.vi"("Refnum in"=w735, "startReg"=u16 220 ("Holding Register"), "Quantity"=u16 4 ("Holding Register"), "Mode"=w734, "Enable"=w728) -> ("Holding Registers"=w733:u16[], "error out"=w727:errorcluster)  [unwired: 6 in, 3 out]
            n443 = Index Array(array=w733) -> (element #1=→"stablePirSP_R":u16, element #2=→"refNoiseSP_R":u16, element #3=→"gasNoiseSP_R":u16, element #4=→"thermoGradientS_R":u16)  [unwired: 4 in]
          }
        }
      }
    }
    n444 = Unbundle By Name(w53) -> ("status"=w44:bool)
    n445 = Not(x=w44) -> (.not. x?=w52:bool)
    n446 = And(x=w44, y=w45) -> (x .and. y?=w46:bool)
    n447 = And(x=w52, y=w45) -> (x .and. y?=→"ConnectionStatus":bool)
    n448 = case shown="True" w46 {
      frame False {
      }
      frame True {
        n449 = local read "Lost"() -> (w59:i16)
        n450 = Increment(x=w59) -> (x+1=→"Lost":i16)
      }
    }
  }
  n451 = case shown="True" w2 {
    tunnel: w1 -> [_ w738]
    frame False {
    }
    frame True {
      n452 = invoke class="VI" method="FP.Close"(reference=w738) -> ()  [unwired: 2 in, 3 out]
    }
  }
